vi "MultiPAS-UV.vi"() -> ()   [LabVIEW 2011]
uses:
  sub/crd/fit/Analysis/analys_meth.ctl
  <vilib>/Analysis/4window.llb/windowTd.ctl
  sub/saveBuildHeader_III.vi
  <vilib>/Utility/file.llb/Write To Spreadsheet File (string).vi
  sub/laserDiagnose_UV.vi
  <vilib>/Instr/_visa.llb/VISA Configure Serial Port (Instr).vi
  sub/QMH/QMH Add Message to Queue (Single Element).vi
  sub/absCalcPlot_UV.vi
  <vilib>/measure/maspectr.llb/FFT Spectrum (Mag-Phase) for 1 Chan.vi
  sub/fftGetMags.vi
  sub/rollingAverage_III.vi
  sub/micUnbundle_III.vi
  sub/pdNormalize_III.vi
  sub/QMH/QMH Add Message to Queue (Array).vi
  <vilib>/measure/NI_MAPro.lvlib
  <vilib>/Analysis/NI_AALPro.lvlib
panel:
  out "working directory":path
  in  "No. Averages":i32=16
  out "saveString":string
  in  "Save Average":bool
  out "Chopper On":bool=TRUE caption="Overtemp"
  in  "Chopper":bool=TRUE
  out "PAS Save":bool caption="Overtemp"
  in  "Data 2":i32[][](array[numeric])=[[-16374, -7248, 2543, 12030, 20279, 26487, 30037, 30583, 28073, 22744, 15131, 5976, -3818, -13288, -21504, -27663, -31155, -31636, -29064, -23686, -16036, -6862, 2936, 12388, 20571, 26684, 30122, 30546, 27911, 22483, 14793, 5595, -4207, -13644, -21795, -27855, -31232, -31591, -28898, -23423, -15695, -6476, 3323, 12743, 20858, 26873, 30194, 30492, 27744, 22213, 14447, 5207, -4597, -14002, -22082, -28044, -31304, -31540, -28731, -23149, -15348, -6093, 3713, 13101, 21145, 27063, 30265, 30442, 27576, 21943, 14103, 4822, -4984, -14354, -22365, -28230, -31373, -31485, -28556, -22876, -14998, -5702, 4104, 13452, 21428, 27245, 30335, 30388, 27400, 21669, 13754, 4435, -5375, -14705, -22643, -28407, -31436, -31426, -28378, -22598, -14648, -5314, 4497, 13803, 21706, 27423, 30394, 30325, 27221, 21390, 13402, 4045, -5763, -15056, -22921, -28586, -31496, -31361, -28198, -22319, -14297, -4924, 4879, 14151, 21982, 27597, 30451, 30257, 27038, 21107, 13050, 3658, -6149, -15402, -23193, -28754, -31546, -31290, -28010, -22033, -13944, -4536, 5266, 14498, 22252, 27767, 30500, 30184, 26849, 20821, 12696, 3267, -6535, -15748, -23462, -28924, -31596, -31216, -27821, -21748, -13587, -4147, 5653, 14838, 22519, 27930, 30549, 30110, 26658, 20535, 12337, 2878, -6919, -16089, -23727, -29087, -31641, -31137, -27627, -21457, -13229, -3753, 6038, 15181, 22786, 28093, 30591, 30031, 26461, 20243, 11979, 2485, -7303, -16428, -23991, -29244, -31678, -31053, -27426, -21159, -12867, -3360, 6424, 15524, 23043, 28252, 30633, 29946, 26262, 19946, 11617, 2096, -7686, -16764, -24246, -29398, -31712, -30964, -27224, -20862, -12503, -2971, 6803, 15859, 23301, 28401, 30661, 29852, 26058, 19648, 11254, 1703, -8069, -17099, -24500, -29547, -31741, -30870, -27018, -20562, -12138, -2575, 7188, 16192, 23556, 28549, 30689, 29756, 25848, 19348, 10891, 1312, -8448, -17430, -24753, -29691, -31765, -30773, -26806, -20259, -11775, -2186, 7566, 16521, 23801, 28690, 30709, 29656, 25634, 19038, 10523, 919, -8831, -17762, -24997, -29833, -31788, -30672, -26593, -19955, -11409, -1792, 7944, 16850, 24047, 28830, 30724, 29548, 25416, 18729, 10152, 523, -9212, -18092, -25245, -29969, -31805, -30566, -26375, -19647, -11041, -1403, 8319, 17173, 24287, 28963, 30734, 29436, 25192, 18418, 9781, 130, -9587, -18413, -25481, -30101, -31814, -30449, -26150, -19332, -10666, -1007, 8697, 17497, 24524, 29090, 30745, 29325, 24968, 18105, 9408, -263, -9962, -18735, -25718, -30228, -31820, -30334, -25921, -19016, -10296, -618, 9072, 17814, 24756, 29213, 30746, 29202, 24738, 17787, 9036, -657, -10338, -19058, -25951, -30350, -31818, -30214, -25690, -18699, -9922, -224, 9442, 18128, 24984, 29330, 30738, 29078, 24502, 17466, 8658, -1050, -10710, -19371, -26178, -30467, -31814, -30088, -25458, -18382, -9550, 167, 9812, 18440, 25206, 29443, 30732, 28947, 24264, 17143, 8281, -1445, -11083, -19685, -26404, -30581, -31807, -29959, -25221, -18059, -9175, 556, 10178, 18750, 25426, 29548, 30718, 28809, 24018, 16812, 7901, -1842, -11457, -19996, -26624, -30690, -31795, -29824, -24980, -17733, -8799, 950, 10549, 19058, 25643, 29655, 30700, 28673, 23773, 16484, 7523, -2235, -11824, -20304, -26840, -30793, -31772, -29682, -24731, -17402, -8415, 1341, 10916, 19363, 25856, 29755, 30677, 28528, 23522, 16151, 7141, -2626, -12191, -20607, -27051, -30891, -31746, -29536, -24481, -17070, -8035, 1733, 11280, 19664, 26064, 29851, 30648, 28381, 23272, 15818, 6762, -3019, -12555, -20906, -27258, -30984, -31717, -29391, -24226, -16736, -7655, 2128, 11641, 19962, 26270, 29940, 30615, 28229, 23013, 15483, 6376, -3409, -12914, -21204, -27459, -31071, -31684, -29236, -23967, -16398, -7271, 2515, 12005, 20258, 26468, 30024, 30577, 28072, 22753, 15143, 5990, -3802, -13276, -21497, -27660, -31157, -31643, -29076, -23707, -16058, -6886, 2908, 12363, 20550, 26666, 30107, 30536, 27914, 22489, 14805, 5607, -4192, -13633, -21787, -27849, -31230, -31597, -28911, -23438, -15716, -6501, 3298, 12719, 20839, 26858, 30182, 30488, 27744, 22223, 14459, 5225, -4579, -13988, -22071, -28040, -31304, -31549, -28743, -23167, -15368, -6113, 3693, 13076, 21126, 27047, 30255, 30438, 27576, 21950, 14113, 4837, -4971, -14340, -22354, -28224, -31375, -31494, -28570, -22895, -15022, -5725, 4080, 13430, 21408, 27230, 30324, 30384, 27402, 21676, 13766, 4449, -5360, -14694, -22636, -28409, -31440, -31436, -28397, -22617, -14674, -5338, 4467, 13781, 21686, 27408, 30385, 30320, 27224, 21398, 13418, 4062, -5748, -15044, -22913, -28584, -31498, -31368, -28212, -22339, -14321, -4948, 4856, 14131, 21963, 27583, 30440, 30254, 27042, 21118, 13062, 3669, -6137, -15390, -23183, -28751, -31551, -31297, -28024, -22049, -13962, -4556, 5245, 14476, 22235, 27754, 30497, 30186, 26857, 20834, 12710, 3283, -6519, -15733, -23453, -28921, -31600, -31226, -27837, -21765, -13610, -4168, 5628, 14820, 22502, 27918, 30540, 30109, 26664, 20544, 12354, 2891, -6906, -16074, -23719, -29085, -31646, -31148, -27642, -21475, -13251, -3777, 6014, 15160, 22765, 28078, 30583, 30027, 26468, 20251, 11994, 2501, -7292, -16415, -23980, -29242, -31682, -31064, -27443, -21181, -12892, -3386, 6397, 15501, 23026, 28238, 30624, 29944, 26269, 19959, 11633, 2110, -7673, -16753, -24239, -29395, -31719, -30974, -27239, -20882, -12528, -2993, 6782, 15835, 23285, 28390, 30651, 29852, 26063, 19660, 11271, 1720, -8053, -17087, -24493, -29546, -31746, -30880, -27031, -20583, -12163, -2599, 7166, 16173, 23538, 28538, 30684, 29758, 25853, 19356, 10906, 1327, -8433, -17416, -24743, -29688, -31769, -30782, -26821, -20280, -11797, -2208, 7543, 16501, 23786, 28680, 30704, 29656, 25642, 19053, 10540, 936, -8814, -17747, -24989, -29827, -31787, -30678, -26606, -19973, -11430, -1817, 7923, 16829, 24031, 28819, 30721, 29552, 25424, 18746, 10174, 543, -9191, -18072, -25231, -29962, -31802, -30567, -26384, -19660, -11057, -1422, 8302, 17159, 24274, 28952, 30738, 29443, 25205, 18435, 9801, 150, -9568, -18401, -25472, -30095, -31811, -30457, -26163, -19349, -10687, -1031, 8679, 17481, 24511, 29082, 30742, 29327, 24979, 18121, 9431, -241, -9943, -18717, -25707, -30221, -31815, -30337, -25930, -19029, -10312, -631, 9058, 17802, 24745, 29207, 30746, 29209, 24750, 17805, 9057, -634, -10316, -19037, -25937, -30340, -31814, -30217, -25700, -18713, -9939, -240, 9429, 18117, 24976, 29328, 30740, 29088, 24519, 17486, 8682, -1027, -10688, -19352, -26164, -30458, -31810, -30091, -25465, -18390, -9561, 154, 9800, 18433, 25201, 29442, 30735, 28959, 24282, 17165, 8308, -1420, -11063, -19665, -26386, -30570, -31801, -29961, -25227, -18068, -9185, 547, 10171, 18745, 25424, 29552, 30726, 28825, 24038, 16835, 7925, -1815, -11429, -19974, -26608, -30681, -31789, -29826, -24984, -17741, -8807, 938, 10536, 19047, 25636, 29657, 30708, 28685, 23794, 16510, 7550, -2205, -11798, -20280, -26821, -30782, -31766, -29684, -24737, -17411, -8429, 1331, 10906, 19356, 25851, 29758, 30684, 28544, 23546, 16178, 7169, -2598, -12162, -20582, -27035, -30879, -31744, -29540, -24485, -17080, -8048, 1721, 11267, 19655, 26061, 29852, 30654, 28395, 23291, 15843, 6786, -2993, -12527, -20884, -27240, -30974, -31713, -29390, -24230, -16744, -7662, 2115, 11635, 19957, 26268, 29945, 30624, 28246, 23035, 15509, 6406, -3382, -12889, -21180, -27444, -31061, -31677, -29236, -23975, -16408, -7284], [-19329, -1252, 17344, 29341, 30145, 19451, 1353, -17227, -29174, -29920, -19175, -1056, 17506, 29408, 30095, 19300, 1159, -17387, -29238, -29860, -19019, -860, 17671, 29475, 30037, 19143, 960, -17553, -29307, -29809, -18866, -664, 17832, 29545, 29987, 18991, 771, -17707, -29365, -29749, -18707, -466, 17992, 29605, 29926, 18832, 570, -17873, -29434, -29694, -18556, -272, 18151, 29670, 29869, 18676, 375, -18031, -29495, -29633, -18395, -75, 18310, 29729, 29809, 18516, 175, -18194, -29561, -29579, -18238, 120, 18469, 29792, 29750, 18362, -17, -18347, -29617, -29515, -18076, 316, 18629, 29848, 29682, 18197, -218, -18510, -29679, -29456, -17921, 513, 18787, 29910, 29626, 18042, -408, -18664, -29734, -29388, -17757, 709, 18941, 29965, 29560, 17875, -609, -18823, -29791, -29326, -17600, 904, 19095, 30023, 29495, 17717, -802, -18975, -29845, -29260, -17434, 1099, 19251, 30075, 29425, 17551, -1001, -19131, -29901, -29194, -17277, 1296, 19408, 30130, 29359, 17393, -1193, -19284, -29953, -29124, -17112, 1491, 19560, 30184, 29290, 17225, -1392, -19440, -30008, -29056, -16949, 1686, 19713, 30237, 29226, 17069, -1581, -19587, -30054, -28982, -16781, 1883, 19866, 30287, 29151, 16898, -1781, -19742, -30107, -28913, -16616, 2079, 20018, 30337, 29082, 16737, -1973, -19888, -30152, -28838, -16449, 2275, 20167, 30383, 29006, 16564, -2174, -20041, -30200, -28765, -16282, 2471, 20321, 30430, 28934, 16403, -2364, -20187, -30243, -28688, -16113, 2669, 20465, 30470, 28853, 16230, -2568, -20341, -30294, -28618, -15953, 2860, 20615, 30519, 28783, 16070, -2755, -20486, -30335, -28537, -15779, 3057, 20760, 30560, 28700, 15892, -2956, -20637, -30378, -28461, -15613, 3252, 20909, 30605, 28628, 15730, -3145, -20777, -30418, -28377, -15440, 3446, 21054, 30645, 28543, 15557, -3345, -20927, -30460, -28299, -15271, 3643, 21199, 30686, 28465, 15391, -3534, -21066, -30495, -28215, -15100, 3839, 21345, 30722, 28380, 15214, -3734, -21213, -30534, -28134, -14928, 4032, 21487, 30760, 28300, 15044, -3926, -21355, -30570, -28052, -14757, 4225, 21627, 30792, 28209, 14870, -4123, -21501, -30607, -27968, -14586, 4419, 21768, 30832, 28129, 14702, -4314, -21637, -30639, -27880, -14413, 4612, 21907, 30859, 28040, 14521, -4515, -21780, -30675, -27796, -14241, 4804, 22048, 30895, 27953, 14352, -4702, -21919, -30705, -27707, -14064, 4999, 22187, 30922, 27859, 14172, -4900, -22060, -30739, -27620, -13892, 5193, 22326, 30954, 27773, 14003, -5090, -22194, -30765, -27524, -13712, 5386, 22462, 30981, 27679, 13823, -5285, -22333, -30794, -27436, -13538, 5580, 22600, 31013, 27591, 13650, -5476, -22466, -30820, -27343, -13363, 5770, 22732, 31033, 27491, 13468, -5673, -22605, -30848, -27251, -13187, 5964, 22870, 31060, 27401, 13292, -5863, -22736, -30870, -27155, -13010, 6156, 23000, 31079, 27299, 13111, -6058, -22873, -30895, -27060, -12833, 6347, 23134, 31104, 27208, 12936, -6248, -23004, -30918, -26965, -12652, 6536, 23260, 31120, 27106, 12753, -6444, -23136, -30939, -26865, -12472, 6729, 23395, 31148, 27011, 12578, -6634, -23266, -30959, -26766, -12296, 6919, 23523, 31161, 26907, 12392, -6830, -23402, -30982, -26665, -12115, 7109, 23652, 31180, 26809, 12213, -7016, -23524, -30992, -26564, -11932, 7301, 23777, 31195, 26704, 12032, -7210, -23655, -31011, -26464, -11755, 7492, 23907, 31211, 26605, 11855, -7395, -23778, -31024, -26358, -11573, 7680, 24031, 31218, 26494, 11665, -7592, -23908, -31039, -26258, -11392, 7871, 24158, 31237, 26394, 11491, -7775, -24031, -31050, -26153, -11210, 8063, 24281, 31247, 26285, 11302, -7972, -24159, -31062, -26046, -11027, 8250, 24407, 31258, 26180, 11124, -8157, -24276, -31067, -25937, -10841, 8438, 24526, 31265, 26071, 10936, -8347, -24401, -31078, -25829, -10659, 8630, 24649, 31275, 25965, 10755, -8533, -24522, -31087, -25721, -10474, 8816, 24770, 31280, 25853, 10566, -8726, -24641, -31091, -25608, -10290, 9003, 24891, 31287, 25746, 10386, -8910, -24756, -31095, -25498, -10105, 9192, 25008, 31287, 25627, 10196, -9102, -24881, -31101, -25386, -9919, 9381, 25127, 31296, 25521, 10019, -9284, -24994, -31099, -25268, -9732, 9570, 25243, 31293, 25403, 9826, -9476, -25113, -31105, -25157, -9544, 9756, 25359, 31298, 25291, 9645, -9655, -25225, -31099, -25040, -9359, 9942, 25473, 31291, 25167, 9453, -9847, -25341, -31102, -24926, -9173, 10124, 25586, 31294, 25057, 9269, -10029, -25450, -31095, -24809, -8986, 10310, 25696, 31284, 24931, 9078, -10218, -25564, -31094, -24688, -8798, 10497, 25812, 31287, 24819, 8896, -10399, -25673, -31085, -24567, -8608, 10682, 25922, 31278, 24698, 8703, -10587, -25785, -31080, -24448, -8422, 10866, 26033, 31274, 24582, 8522, -10765, -25890, -31067, -24321, -8230, 11050, 26140, 31263, 24455, 8325, -10952, -26001, -31064, -24201, -8040, 11234, 26248, 31255, 24338, 8142, -11132, -26106, -31054, -24079, -7852, 11417, 26353, 31243, 24207, 7948, -11316, -26217, -31041, -23952, -7662, 11601, 26464, 31236, 24089, 7763, -11494, -26315, -31025, -23829, -7471, 11782, 26562, 31217, 23957, 7567, -11682, -26422, -31014, -23702, -7282, 11962, 26667, 31205, 23834, 7383, -11859, -26521, -30998, -23575, -7092, 12144, 26770, 31187, 23704, 7186, -12043, -26626, -30981, -23444, -6900, 12328, 26875, 31176, 23582, 7003, -12218, -26724, -30962, -23316, -6709, 12505, 26971, 31154, 23446, 6805, -12401, -26825, -30946, -23189, -6517, 12687, 27073, 31139, 23322, 6620, -12576, -26919, -30922, -23054, -6323, 12867, 27170, 31114, 23185, 6422, -12760, -27022, -30904, -22923, -6132, 13047, 27272, 31096, 23060, 6237, -12934, -27114, -30879, -22790, -5940, 13222, 27362, 31068, 22921, 6041, -13116, -27212, -30855, -22657, -5748, 13401, 27461, 31048, 22790, 5853, -13289, -27302, -30828, -22522, -5555, 13577, 27549, 31019, 22652, 5652, -13472, -27398, -30806, -22388, -5362, 13753, 27645, 30995, 22521, 5463, -13642, -27487, -30776, -22248, -5169, 13928, 27733, 30963, 22376, 5266, -13823, -27584, -30750, -22113, -4975, 14106, 27828, 30937, 22246, 5082, -13992, -27669, -30717, -21974, -4782, 14280, 27914, 30902, 22101, 4880, -14174, -27760, -30689, -21837, -4588, 14454, 28006, 30875, 21965, 4692, -14340, -27843, -30653, -21693, -4391, 14631, 28092, 30840, 21822, 4494, -14519, -27934, -30620, -21552, -4198, 14805, 28179, 30808, 21688, 4308, -14687, -28015, -30582, -21410, -4004, 14975, 28262, 30770, 21540, 4106, -14861, -28103, -30548, -21268, -3808, 15149, 28349, 30739, 21402, 3916, -15032, -28183, -30512, -21124, -3614, 15319, 28430, 30697, 21255, 3715, -15205, -28267, -30475, -20982, -3421, 15490, 28513, 30664, 21116, 3524, -15376, -28348, -30435, -20837, -3225, 15660, 28592, 30617, 20962, 3327, -15550, -28432, -30397, -20695, -3032, 15829, 28673, 30581, 20820, 3134, -15711, -28506, -30353, -20546, -2837, 15994, 28746, 30530, 20669, 2933, -15887, -28585, -30311, -20400, -2641, 16167, 28828, 30496, 20528, 2745, -16052, -28660, -30264, -20248, -2445, 16335, 28901, 30445, 20376, 2544, -16221, -28737, -30219, -20102, -2250, 16505, 28983, 30406, 20231, 2357, -16381, -28808, -30171, -19950, -2053, 16670, 29053, 30355, 20075, 2154, -16552, -28883, -30127, -19803, -1859, 16835, 29128, 30308, 19930, 1965, -16714, -28952, -30073, -19650, -1663, 17001, 29192, 30255, 19772, 1764, -16881, -29028, -30026, -19496, -1467, 17165, 29268, 30208, 19626, 1572, -17043, -29095, -29977, -19346]]
  out "Filtering":bool caption="Time has Elapsed"
  in  "Switch Filter":bool
  in  "Auto Filter":bool
  out "Elapsed Time (min)":dbl caption="Elapsed Time (s)" format="%#.1g"
  in  "Filter Length (min)":dbl=6.0 caption="Time Target (s)"
  in  "Sample Length (min)":dbl=24.0 caption="Time Target (s)" format="%#.1f"
  out "Time has Elapsed":bool
  in  "Time Target (s)":dbl=1.0
  in  "All Emit":bool
  in  "Alignment Mode":bool
  in  "445 Emission":bool
  in  "445 Power (mW)":dbl(slide)=75.0 min=0.0 max=75.0 step=1.0 scale=0.0..75.0
  in  "375 Emission":bool
  in  "375 Power (mW)":dbl(slide)=100.0 min=0.0 max=50.0 step=1.0 scale=0.0..50.0
  in  "320 Emission":bool=TRUE
  out "Overtemp":bool
  in  "Tab Control":T1(tab)=enum."Oscilloscope"
  out "Laser Currents":T2(graph)
  in  "Chopper Port":refnum<visa-resource-name>="COM6"
  out "sweeps":path caption="Microphone File Path"
  in  "save interval (ms)":u32=1000
  out "Error Console":T3
  out "pas":path caption="Microphone File Path"
  out "Laser Temperatures":T2(graph)
  in  "pd id":u32=2
  in  "mic id":u32
  in  "mic cal, scu":dbl=5.41531278804282e-05 format="%#_3e"
  in  "mic cal, scu":dbl=5.59307241877627e-05 format="%#_3e"
  in  "320 Port":refnum<visa-resource-name>="COM7"
  in  "375 Port":refnum<visa-resource-name>="COM8"
  in  "445 Port":refnum<visa-resource-name>="COM9"
  in  "Teensy Port":refnum<visa-resource-name>="COM10"
  in  "Save Data":bool
  in  "405 PD Cal 3":dbl=0.0075
  in  "532 PD Cal 3":dbl=0.0861
  in  "660 PD Cal 3":dbl=0.005
  out "Laser Powers":T2(graph)
  in  "tau Rolling Avg":i32=8
  out "error out":errorcluster
  in  "Channel B Settings":T4={"Enabled"=TRUE, "Coupling"=1, "Range"=8, "Analogue Offset"=0.0} {"Range" items=["20 mV"=1, "50 mV"=2, "100 mV"=3, "200 mV"=4, "500 mV"=5, "1 V"=6, "2 V"=7, "5 V"=8, "10 V"=9, "20 V"=10]; "Coupling" items=["AC", "DC"]}
  in  "Rapid Block Acquisition Settings":T5={"preTriggerSamples"=0, "postTriggerSamples"=45000, "timebase"=1, "Down-Sample Mode"=4, "Down Sample Ratio"=10, "Oversample"=1, "Number of Captures"=100} {"Down Sample Ratio" min=1 step=1; "Down-Sample Mode" items=["None"=0, "Aggregate"=1, "Decimate"=2, "Average"=4]}
  in  "crd delay":u32=1000
  in  "Trigger Settings":T6={"Trigger Enabled"=TRUE, "Trigger Source"=enum."Channel B", "Trigger Threshold (Volts)"=1.0, "Trigger Direction"=3, "Trigger Delay (samples)"=0, "Auto Trigger Time (ms)"=1000} {"Trigger Direction" items=["Rising"=2, "Falling"=3]}
  in  "Channel A Settings":T4={"Enabled"=TRUE, "Coupling"=0, "Range"=3, "Analogue Offset"=0.0} {"Range" items=["20 mV"=1, "50 mV"=2, "100 mV"=3, "200 mV"=4, "500 mV"=5, "1 V"=6, "2 V"=7, "5 V"=8, "10 V"=9, "20 V"=10]; "Coupling" items=["AC", "DC"]}
  in  "factor":sgl=10.0
  in  "N":i32=4400
  in  "sweep":bool
  out "freqscan":cluster{i32[], "Best Gaussian Fit":dbl[]}[](graph) caption="Frequency Sweep"
  out "sweep progress":dbl(slide) scale=0.0..1.0
  in  "Autosweep?":bool=TRUE
  in  "set freqs":bool
  out "Calculated Resonance (Hz)":dbl=1370.0
  in  "Data Start Frequency (Hz)":i32=1355
  in  "Data End Frequency (Hz)":i32=1405
  in  "320 F (Hz)":i32=1368
  in  "375 F (Hz)":i32=1372
  in  "445 F (Hz)":i32=1370
  in  "Chart Rolling Average":i32=16
  out "pdwave":waveform(i32)(graph) caption="Photodiode Waveform"
  out "pd ts":cluster{dbl, dbl, dbl}(graph)
  out "pdfft":cluster{"f0":dbl, "df":dbl, "magnitude":dbl[]}(graph) caption="Photodiode FFT"
  in  "rollavg":i32=16 caption="Dispaly Averaging (Transfers to Absorption Data!)"
  out "mic ts":T7(graph)
  out "micfft":cluster{"f0":dbl, "df":dbl, "magnitude":dbl[]}(graph) caption="Photodiode FFT"
  out "micwave":waveform(i32)(graph) caption="Photodiode Waveform"
  in  "tau0":dbl
  in  "getbkg":bool
  out "AAE":dbl(graph)
  in  "Bkg Values (mV)":cluster{dbl, dbl, dbl}
  out "Absorption Spectrum":cluster{dbl[], "Best Power Fit":dbl[]}[](graph)
  in  "cellcal":dbl=95000.0 caption="Cell Calibration Coefficient (mV/mW)"
  out "abs/ext":cluster{dbl, dbl, dbl, "b_ext (1/Mm)":dbl}(graph)
  out "tau":dbl(graph)
  out "decay":cluster{i32, sgl, dbl[]}[](graph)
  out "residual":cluster{i32, sgl, dbl[]}(graph)
  out "Status":string
  in  "Exit":bool
  in  "State Variables":cluster{"CurrentFile":path}
  # "MultiPAS-UV | AeroSmith Labs (2017)"
  # "Laser Control"
  # "Filter Control"
  # "Communications"
  # "Sound Card Parameters"
  # "Data File Options"
  # "File paths are populated automatically at <...\\My Documents\\MultiPAS Data\\>.  To save in another location, turn on \"Save Data\" and follow the prompts to choose an alternate working directory."
  # "Photodiode Calibration"
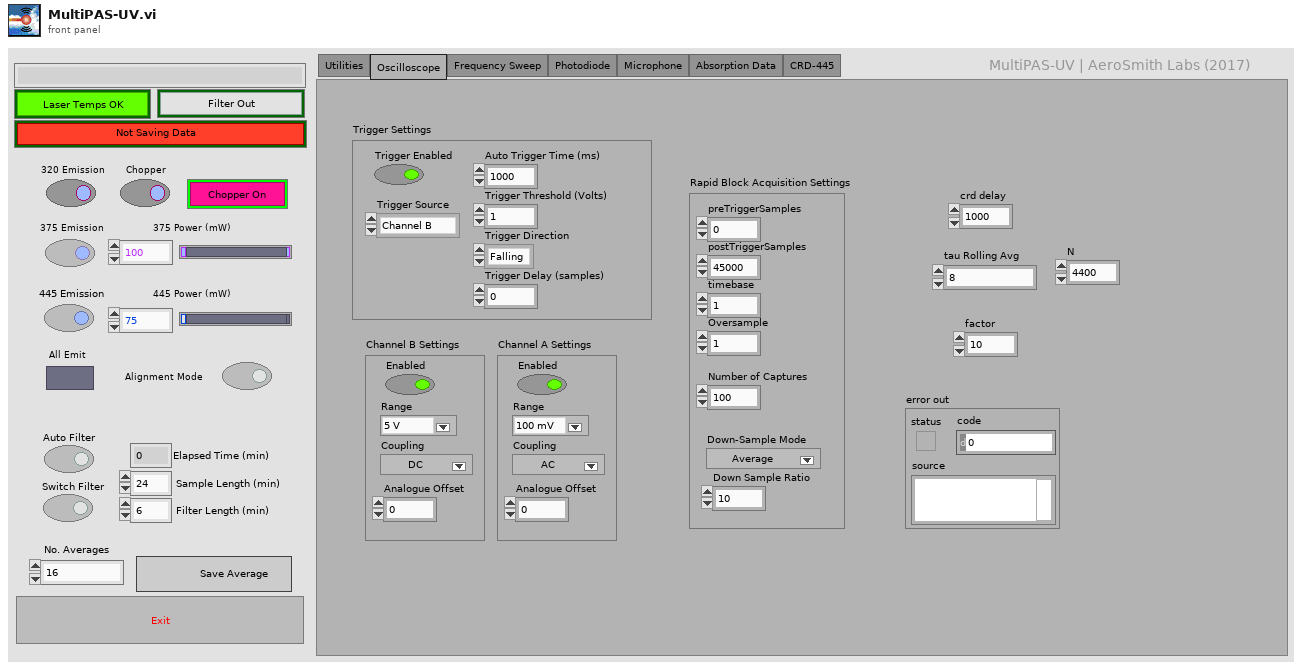
[diagram p1: front panel]
types:
  T1 = enum32{"Utilities", "Oscilloscope", "Frequency Sweep", "Photodiode", "Microphone", "Absorption Data", "CRD-445"}
  T2 = cluster{"Temp (C)":dbl, "Temp (C)":dbl, "Temp (C)":dbl}
  T3 = cluster{"status":bool, "code":i32, "Message":string}
  T4 = cluster{"Enabled":bool, "Coupling":i16, "Range":u16, "Analogue Offset":sgl}
  T5 = cluster{"preTriggerSamples":u32, "postTriggerSamples":u32, "timebase":u32, "Down-Sample Mode":i32, "Down Sample Ratio":u32, "Oversample":i16, "Number of Captures":u32}
  T6 = cluster{"Trigger Enabled":bool, "Trigger Source":enum16{"Channel A", "Channel B", "Channel C", "Channel D", "Ext."}, "Trigger Threshold (Volts)":dbl, "Trigger Direction":u16, "Trigger Delay (samples)":u32, "Auto Trigger Time (ms)":i16}
  T7 = cluster{"422 Mean":dbl, "532 Mean":dbl, "785 Mean":dbl}
  T8 = cluster{"# buffers":i32, "Buffer size":i32, "unit (ms)":enum16{"time (ms)", "Samples"}}
  T9 = typedef "SoundHandle.ctl" = cluster{"DeviceID":u16, "Samples/buf":u32, "Sampl rate":u32, "Bits/sample":u16, "Channels":u8, "Opened":bool}
  T10 = cluster{"Output Power at Laser Head":dbl, "Output Power at Laser Head":dbl, "Output Power at Laser Head":dbl}
  T11 = cluster{"Current (mA)":dbl, "Current (mA)":dbl, "Current (mA)":dbl}
  T12 = cluster{"405 Mean":dbl, "532 Mean":dbl, "660 Mean":dbl}
  T13 = typedef "NI_AALPro.lvlib/windowTd.ctl" = u32
  T14 = cluster{"785 New Array":dbl[], "785 Mean":dbl, "785 SD":dbl}
  T15 = cluster{"532 New Array":dbl[], "532 Mean":dbl, "532 SD":dbl}
  T16 = cluster{"422 New Array":dbl[], "422 Mean":dbl, "422 SD":dbl}
  T17 = typedef "analys_meth.ctl" = enum16{"DFT-1", "DFT-5", "LRS"}
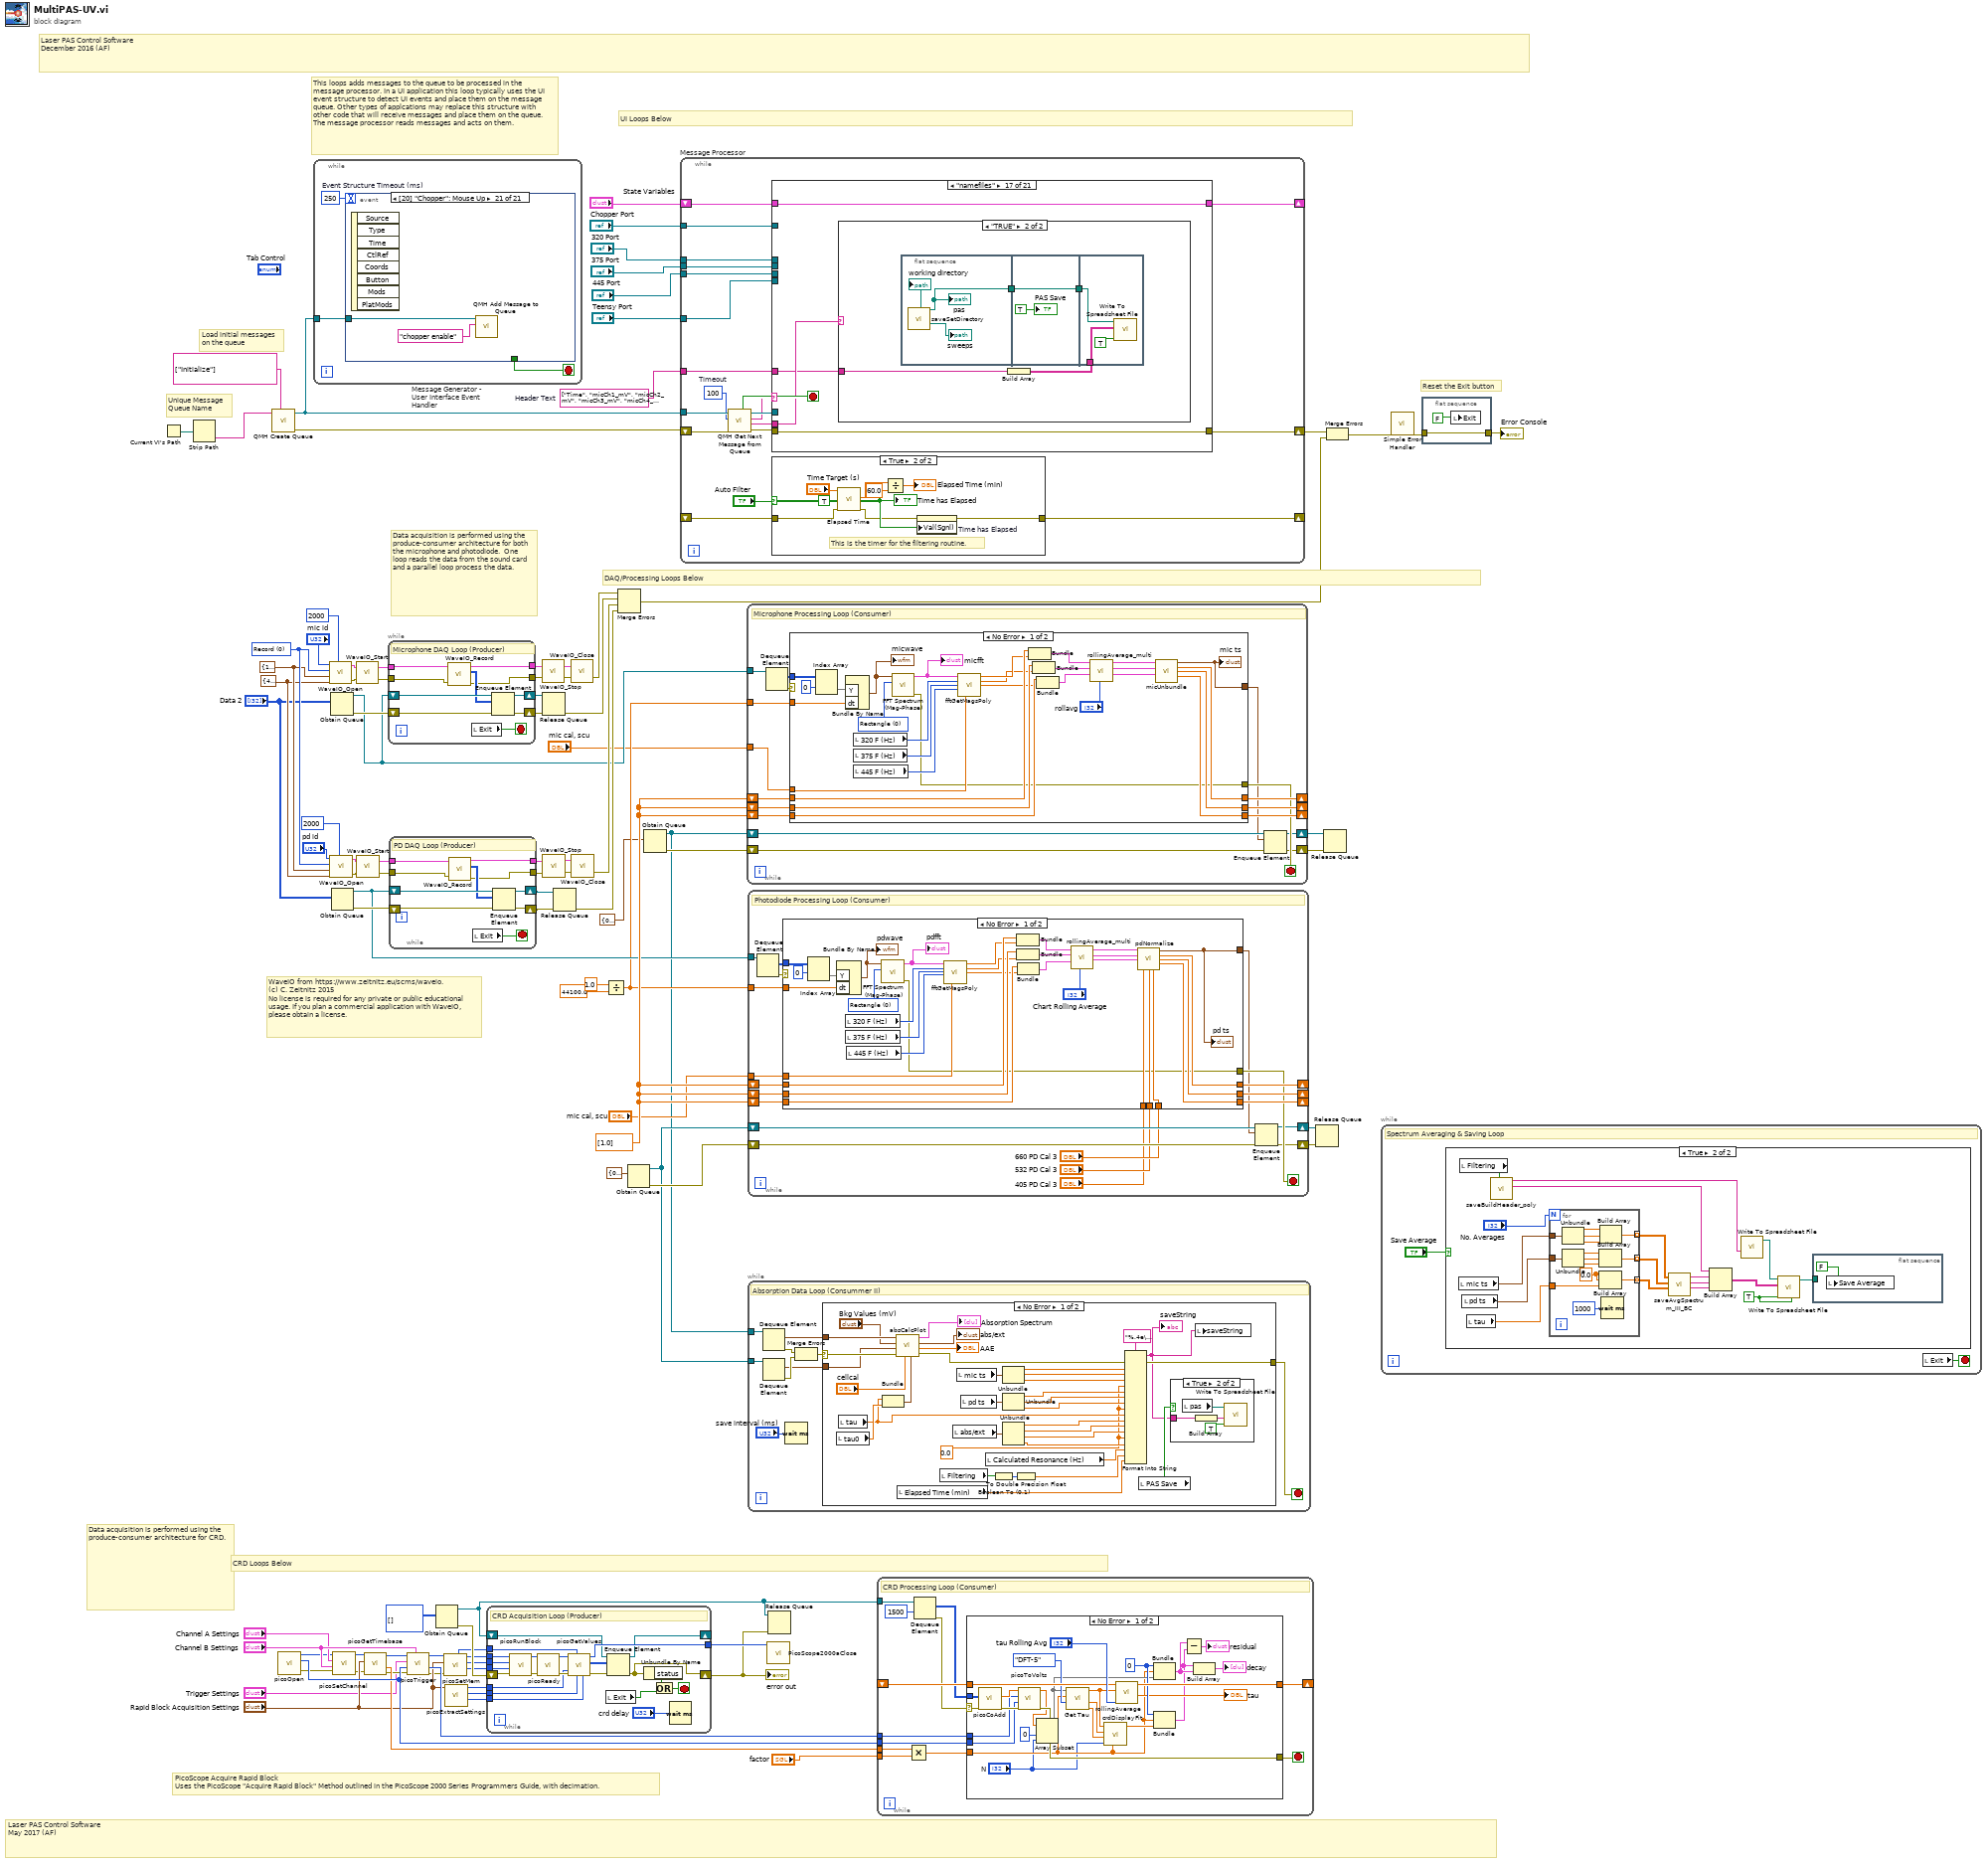
[diagram p0: block diagram]
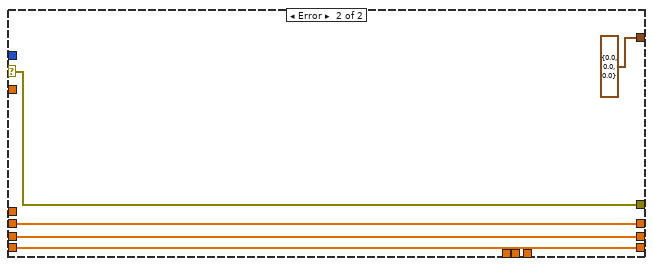
[diagram p6: hidden frame]
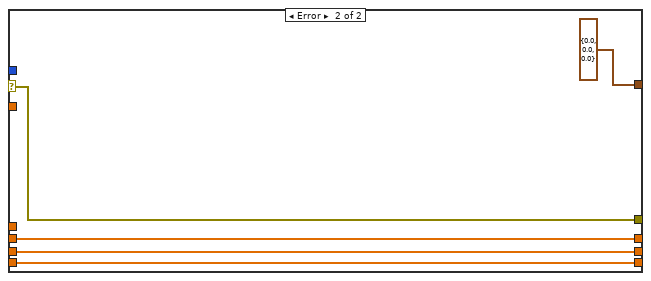
[diagram p7: hidden frame]
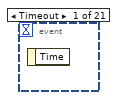
[diagram p8: hidden frame]
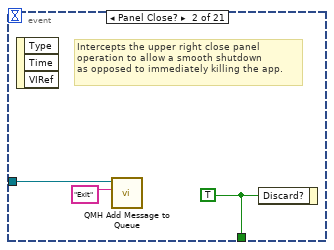
[diagram p9: hidden frame]
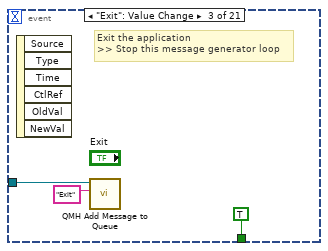
[diagram p10: hidden frame]
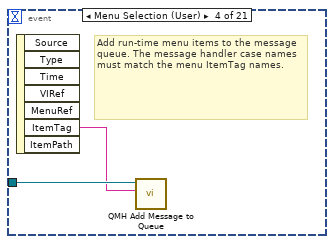
[diagram p11: hidden frame]
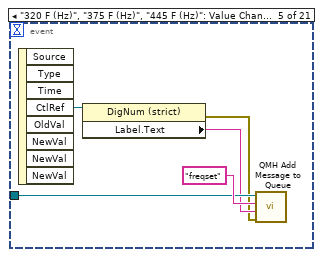
[diagram p12: hidden frame]
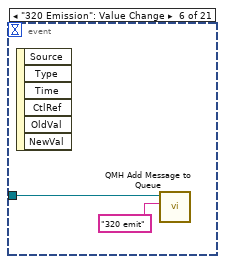
[diagram p13: hidden frame]
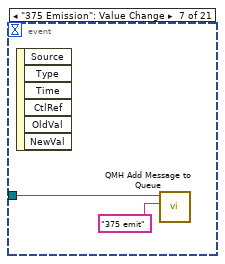
[diagram p14: hidden frame]
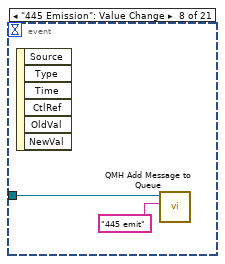
[diagram p15: hidden frame]
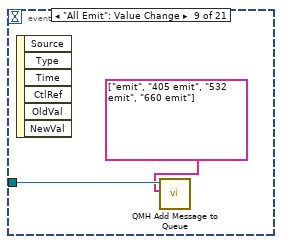
[diagram p16: hidden frame]
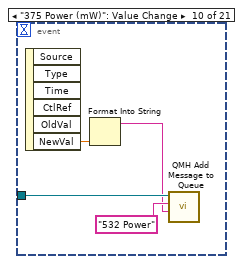
[diagram p17: hidden frame]
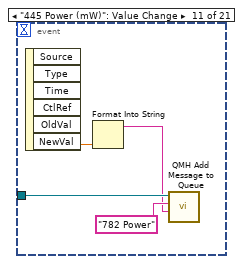
[diagram p18: hidden frame]
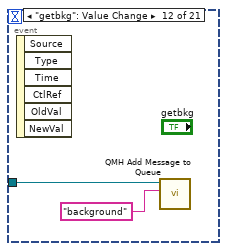
[diagram p19: hidden frame]
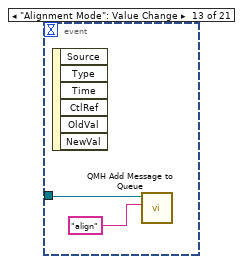
[diagram p20: hidden frame]
diagram:
  w30 = string[] ["Time", "micCh1_mV", "micCh2_mV", "micCh3_mV", "micCh4_mV", "pdCh1_mV", "pdCh2_mV", "pdCh3_mV", "pdCh4_mV", "tau_sec", "babsCh1_Mm", "babsCh2_Mm", "babsCh3_Mm", "babsCh4_Mm", "bext_Mm", "fres_Hz", "filter_state", "elapsedTime_min"]  # Header Text
  w50 = T8 {"# buffers"=10, "Buffer size"=44100, "unit (ms)"=enum."Samples"} ("Buffer")
  w49 = cluster{"Rate":i32, "Bits":i32, "Channels":i32} {"Rate"=44100, "Bits"=24, "Channels"=2} ("Format")
  w51 = u16 0 items=["Record", "Play", "Loopback", "ASIO input", "ASIO output"] ("Direction (Record)")
  w81 = dbl[] [1.0] ("X")
  # "PicoScope Acquire Rapid Block\nUses the PicoScope \"Acquire Rapid Block\" Method outlined in the PicoScope 2000 Series Programmers Guide, with decimation."
  # "Data acquisition is performed using the produce-consumer architecture for CRD."
  # "CRD Loops Below"
  # "Laser PAS Control Software\nMay 2017 (AF)"
  # "Laser PAS Control Software\nDecember 2016 (AF)"
  # "Data acquisition is performed using the produce-consumer architecture for both the microphone and photodiode.  One loop reads the data from the sound card and a parallel loop process the data."
  # "WaveIO from https://www.zeitnitz.eu/scms/waveio.\n(c) C. Zeitnitz 2015\nNo license is required for any private or public educational usage. If you plan a commercial application with WaveIO, please obtain a license."
  # "This loops adds messages to the queue to be processed in the message processor. In a UI application this loop typically uses the UI event structure to detect UI events and place them on the message queue. Other types of applcations may replace this structure with other code that will receive messages and place them on the queue.  The message processor reads messages and acts on them."
  # "Reset the Exit button"
  # "Unique Message\nQueue Name"
  # "Load initial messages\non the queue"
  # "DAQ/Processing Loops Below"
  # "UI Loops Below"
  n1 = Current VI's Path() -> (path=w96:path)
  n2 = Strip Path(path=w96) -> (name=w97:string)  [unwired: 1 out]
  n3 = call "QMH Create Queue.vi"("Initial Messages"=string[] ["Initialize"], "Message queue name (unnamed)"=w97) -> ("error out"=w93:errorcluster, "queue out"=w78:refnum<queue>)  [unwired: 8 in]
  n4 = call "picoOpen.vi"() -> ("error out"=w5:errorcluster, "maxADC"=w24:i16, "Handle Out"=w4:i16)  [unwired: 8 in, 1 out]
  n5 = while "Message Generator - User Interface Event Handler" {
    tunnel: w78 -> [w98]
    stop <- w99 stop-if-true
    w100 = 250  # Event Structure Timeout (ms)
    n6 = event shown="[20] \"Chopper\": Mouse Up" {
      selector: _ -> [_ _ _ _ _ _ _ _ _ _ _ _ _ _ _ _ _ _ _ _ _]
      dyn-events: _ -> [_ _ _ _ _ _ _ _ _ _ _ _ _ _ _ _ _ _ _ _ _]
      timeout: w100 -> [_ _ _ _ _ _ _ _ _ _ _ _ _ _ _ _ _ _ _ _ _]
      tunnel: [_ w103 TRUE ("Discard?") _ _ _ _ _ _ _ _ _ _ _ _ _ _ _ _ _ _] -> w99
      tunnel: w98 -> [_ w102 w105 w108 w112 w114 w116 w118 w121 w124 w128 w130 w132 w135 w139 w144 w149 w153 w158 w160 w162]
      event Timeout {
        n7 = event-data() -> ()  [unwired: 1 in, 1 out]
      }
      event Panel Close? {
        w103 = TRUE ("Discard?")
        # "Intercepts the upper right close panel\noperation to allow a smooth shutdown\nas opposed to immediately killing the app."
        n8 = event-data() -> ()  [unwired: 1 in, 3 out]
        n9 = call-poly "QMH Add Message to Queue.vi"("Message"="Exit", "queue in"=w102) -> ()  [unwired: 8 in, 2 out]
        n10 = event-data("Discard?"=w103) -> ()  [unwired: 1 in, 1 out]
      }
      event "Exit": Value Change {
        # "Exit the application\n>> Stop this message generator loop"
        n11 = event-data() -> ()  [unwired: 1 in, 6 out]
        n12 = call-poly "QMH Add Message to Queue.vi"("Message"="Exit", "queue in"=w105) -> ()  [unwired: 8 in, 2 out]
      }
      event Menu Selection (User) {
        # "Add run-time menu items to the message\nqueue. The message handler case names must match the menu ItemTag names."
        n13 = event-data() -> ("ItemTag"=w107:string)  [unwired: 1 in, 6 out]
        n14 = call-poly "QMH Add Message to Queue.vi"("Message"=w107, "queue in"=w108) -> ()  [unwired: 8 in, 2 out]
      }
      event "320 F (Hz)", "375 F (Hz)", "445 F (Hz)": Value Change {
        n15 = event-data() -> ("CtlRef"=w111:refnum<vi>)  [unwired: 1 in, 7 out]
        n16 = property class="DigNum (strict)"(reference=w111) -> (error out=w109:errorcluster, "Label.Text"=w110:string)  [unwired: 1 in, 1 out]
        n17 = call-poly "QMH Add Message to Queue.vi"("error in (no error)"=w109, "Parameter"=w110, "Message"="freqset", "queue in"=w112) -> ()  [unwired: 6 in, 2 out]
      }
      event "320 Emission": Value Change {
        n18 = event-data() -> ()  [unwired: 1 in, 6 out]
        n19 = call-poly "QMH Add Message to Queue.vi"("Message"="320 emit", "queue in"=w114) -> ()  [unwired: 8 in, 2 out]
      }
      event "375 Emission": Value Change {
        n20 = event-data() -> ()  [unwired: 1 in, 6 out]
        n21 = call-poly "QMH Add Message to Queue.vi"("Message"="375 emit", "queue in"=w116) -> ()  [unwired: 8 in, 2 out]
      }
      event "445 Emission": Value Change {
        n22 = event-data() -> ()  [unwired: 1 in, 6 out]
        n23 = call-poly "QMH Add Message to Queue.vi"("Message"="445 emit", "queue in"=w118) -> ()  [unwired: 8 in, 2 out]
      }
      event "All Emit": Value Change {
        n24 = event-data() -> ()  [unwired: 1 in, 6 out]
        n25 = call-poly "QMH Add Message to Queue.vi"("Messages"=string[] ["emit", "405 emit", "532 emit", "660 emit"], "queue in"=w121) -> ()  [unwired: 8 in, 2 out]
      }
      event "375 Power (mW)": Value Change {
        n26 = event-data() -> ("NewVal"=w123:dbl)  [unwired: 1 in, 5 out]
        n27 = Format Into String(w123) -> (resulting string=w122:string)  [unwired: 3 in, 1 out]
        n28 = call-poly "QMH Add Message to Queue.vi"("Parameter"=w122, "Message"="532 Power", "queue in"=w124) -> ()  [unwired: 7 in, 2 out]
      }
      event "445 Power (mW)": Value Change {
        n29 = event-data() -> ("NewVal"=w127:dbl)  [unwired: 1 in, 5 out]
        n30 = Format Into String(w127) -> (resulting string=w126:string)  [unwired: 3 in, 1 out]
        n31 = call-poly "QMH Add Message to Queue.vi"("Parameter"=w126, "Message"="782 Power", "queue in"=w128) -> ()  [unwired: 7 in, 2 out]
      }
      event "getbkg": Value Change {
        n32 = event-data() -> ()  [unwired: 1 in, 6 out]
        n33 = call-poly "QMH Add Message to Queue.vi"("Message"="background", "queue in"=w130) -> ()  [unwired: 8 in, 2 out]
      }
      event "Alignment Mode": Value Change {
        n34 = event-data() -> ()  [unwired: 1 in, 6 out]
        n35 = call-poly "QMH Add Message to Queue.vi"("Message"="align", "queue in"=w132) -> ()  [unwired: 8 in, 2 out]
      }
      event "sweep": Value Change {
        n36 = event-data() -> ()  [unwired: 1 in, 6 out]
        n37 = call-poly "QMH Add Message to Queue.vi"("Message"="sweep", "queue in"=w135) -> ()  [unwired: 8 in, 2 out]
      }
      event "set freqs": Value Change {
        n38 = event-data() -> ()  [unwired: 1 in, 6 out]
        n39 = local read "Calculated Resonance (Hz)"() -> (w138:dbl)
        n40 = Format Into String(w138) -> (resulting string=w137:string, error out=w136:errorcluster)  [unwired: 3 in]
        n41 = call-poly "QMH Add Message to Queue.vi"("error in (no error)"=w136, "Parameter"=w137, "Message"="setfreqs", "queue in"=w139) -> ()  [unwired: 6 in, 2 out]
      }
      event "Save Data": Value Change {
        n42 = event-data() -> ("NewVal"=w143:bool)  [unwired: 1 in, 5 out]
        n43 = Format Into String(w143) -> (resulting string=w142:string, error out=w141:errorcluster)  [unwired: 3 in]
        n44 = call-poly "QMH Add Message to Queue.vi"("error in (no error)"=w141, "Parameter"=w142, "Message"="namefiles", "queue in"=w144) -> ()  [unwired: 6 in, 2 out]
      }
      event "Switch Filter": Value Change {
        n45 = event-data() -> ("NewVal"=w148:bool)  [unwired: 1 in, 5 out]
        n46 = local write "Filtering"(w148) -> ()
        n47 = Format Into String(w148) -> (resulting string=w146:string)  [unwired: 3 in, 1 out]
        n48 = call-poly "QMH Add Message to Queue.vi"("Parameter"=w146, "Message"="filterswitch", "queue in"=w149) -> ()  [unwired: 7 in, 2 out]
      }
      event "Time has Elapsed": Value Change {
        n49 = event-data() -> ("NewVal"=w152:bool)  [unwired: 1 in, 5 out]
        n50 = local read "Filtering"() -> (w151:bool)
        n51 = call "filterCreateMsg.vi"("time elapsed?"=w152, "auto sweep (true)"="Autosweep?", "filtering (true)"=w151, "queue in"=w153) -> ()  [unwired: 6 in, 2 out]
      }
      event "Calculated Resonance (Hz)": Value Change {
        n52 = event-data() -> ("NewVal"=w156:dbl)  [unwired: 1 in, 5 out]
        n53 = Format Into String(w156) -> (resulting string=w154:string, error out=w155:errorcluster)  [unwired: 3 in]
        n54 = call-poly "QMH Add Message to Queue.vi"("error in (no error)"=w155, "Parameter"=w154, "Message"="setfreqs", "queue in"=w158) -> ()  [unwired: 6 in, 2 out]
      }
      event "PAS Save": Value Change {
        n55 = event-data() -> ()  [unwired: 1 in, 6 out]
        n56 = call-poly "QMH Add Message to Queue.vi"("Message"="setwd", "queue in"=w160) -> ()  [unwired: 8 in, 2 out]
      }
      event "Chopper": Mouse Up {
        n57 = event-data() -> ()  [unwired: 1 in, 8 out]
        n58 = call-poly "QMH Add Message to Queue.vi"("Message"="chopper enable", "queue in"=w162) -> ()  [unwired: 8 in, 2 out]
      }
    }
  }
  n59 = call <userlib>:"WaveIO_Open.vi"("idev"="mic id", "Watchdog timeout (msec) (default=OFF)"=2000, "device type (Record)"=w51, "Buffer Config"=w50, "Format (44kHz, 16Bit, stereo)"=w49) -> ("Sound Handle Out"=w75:T9, "error out"=w74:errorcluster)  [unwired: 2 in]
  n60 = call <userlib>:"WaveIO_Open.vi"("idev"="pd id", "Watchdog timeout (msec) (default=OFF)"=2000, "device type (Record)"=w51, "Buffer Config"=w50, "Format (44kHz, 16Bit, stereo)"=w49) -> ("Sound Handle Out"=w59:T9, "error out"=w60:errorcluster)  [unwired: 2 in]
  n61 = Obtain Queue(element data type="Data 2") -> (queue out=w43:refnum<queue>, error out=w82:errorcluster)  [unwired: 4 in, 1 out]
  n62 = Obtain Queue(element data type="Data 2") -> (queue out=w47:refnum<queue>, error out=w56:errorcluster)  [unwired: 4 in, 1 out]
  n63 = call "picoSetChannel.vi"("error in (no error)"=w5, "Channel B Settings"="Channel B Settings", "Channel A Settings"="Channel A Settings", "Handle Out"=w4) -> ("error out"=w16:errorcluster, "Handle Out"=w19:i16)  [unwired: 6 in]
  n64 = call <userlib>:"WaveIO_Start.vi"("error in (no error)"=w74, "Handle"=w75) -> ("error out"=w72:errorcluster, "Handle Out"=w73:T9)
  n65 = call <userlib>:"WaveIO_Start.vi"("error in (no error)"=w60, "Handle"=w59) -> ("error out"=w62:errorcluster, "Handle Out"=w61:T9)
  n66 = call "picoGetTimebase.vi"("error in (no error)"=w16, "Rapid Block Acquisition Settings"="Rapid Block Acquisition Settings", "handle in"=w19) -> ("error out"=w17:errorcluster, "Sample Interval"=w23:sgl, "handle out"=w18:i16)  [unwired: 6 in]
  n67 = while {
    shift-right: [w171] -> w83
    shift-left: w43 -> [w169]
    shift-right: [w172] -> w84
    shift-left: w82 -> [w170]
    tunnel: w73 -> [w167]
    tunnel: w72 -> [w166]
    tunnel: [w164] -> w69
    tunnel: [w163] -> w68
    stop <- w168 stop-if-true
    # "Microphone DAQ Loop (Producer)"
    n68 = call <userlib>:"WaveIO_Record.vi"("Handle"=w167, "error in (no error)"=w166) -> ("Handle Out"=w164:T9, "Data"=w165:i32[][], "error out"=w163:errorcluster)  [unwired: 1 in, 2 out]
    n69 = local read "Exit"() -> (w168:bool)
    n70 = Enqueue Element(queue=w169, element=w165, error in (no error)=w170) -> (queue out=w171:refnum<queue>, error out=w172:errorcluster)  [unwired: 1 in, 1 out]
  }
  n71 = while {
    shift-right: [w181] -> w55
    shift-left: w47 -> [w179]
    shift-right: [w182] -> w54
    shift-left: w56 -> [w180]
    tunnel: w61 -> [w177]
    tunnel: w62 -> [w176]
    tunnel: [w174] -> w65
    tunnel: [w173] -> w66
    stop <- w178 stop-if-true
    # "PD DAQ Loop (Producer)"
    n72 = call <userlib>:"WaveIO_Record.vi"("Handle"=w177, "error in (no error)"=w176) -> ("Handle Out"=w174:T9, "Data"=w175:i32[][], "error out"=w173:errorcluster)  [unwired: 1 in, 2 out]
    n73 = local read "Exit"() -> (w178:bool)
    n74 = Enqueue Element(queue=w179, element=w175, error in (no error)=w180) -> (queue out=w181:refnum<queue>, error out=w182:errorcluster)  [unwired: 1 in, 1 out]
  }
  n75 = call "picoTrigger.vi"("Trigger Channel Settings"="Channel B Settings", "error in (no error)"=w17, "maxADC"=w24, "Trigger Settings"="Trigger Settings", "Handle In"=w18) -> ("error out"=w10:errorcluster, "Range"=w25:u16, "handle out"=w11:i16)  [unwired: 4 in]
  n76 = Obtain Queue(element data type=i16[][] [] ("buffer")) -> (queue out=w1:refnum<queue>, error out=w29:errorcluster)  [unwired: 4 in, 1 out]
  n77 = call "picoSetMem.vi"("error in (no error)"=w10, "Rapid Block Acquisition Settings"="Rapid Block Acquisition Settings", "Handle In"=w11) -> ("timebase"=w8:u32, "postTriggerSamples"=w7:u32, "Handle Out"=w6:i16, "nCaptures"=w9:u16)  [unwired: 4 in, 1 out]
  n78 = call "picoExtractSettings.vi"("Rapid Block Acquisition Settings"="Rapid Block Acquisition Settings") -> ("Down-Sample Mode"=w15:i32, "Down Sample Ratio"=w14:u32, "Numeric"=w13:i32)  [unwired: 8 in]
  n79 = while {
    tunnel: w6 -> [w200]
    tunnel: w7 -> [w199]
    tunnel: w8 -> [w198]
    tunnel: w9 -> [w204]
    tunnel: w13 -> [w196]
    tunnel: w14 -> [w195]
    tunnel: w15 -> [w194]
    tunnel: [w189] -> w28
    shift-right: [w186] -> _
    shift-left: w1 -> [w187]
    shift-right: [w184] -> w2
    shift-left: w29 -> [w183]
    stop <- w193 stop-if-true
    # "CRD Acquisition Loop (Producer)"
    n80 = call "picoRunBlock.vi"("error in (no error)"=w183, "timebase"=w198, "postTriggerSamples"=w199, "Handle In"=w200) -> ("error out"=w203:errorcluster, "handle"=w202:i16)  [unwired: 5 in, 1 out]
    n81 = call "picoReady.vi"("error in (no error)"=w203, "handle in"=w202) -> ("error out"=w201:errorcluster, "handle out"=w197:i16)  [unwired: 8 in]
    n82 = call "picoGetValues.vi"("Down-Sample Mode"=w194, "Down Sample Ratio"=w195, "nCaptures"=w204, "error in (no error)"=w201, "postTriggerSamples"=w196, "Handle In"=w197) -> ("error out"=w185:errorcluster, "buffer"=w188:i16[][], "handle"=w189:i16)  [unwired: 3 in]
    n83 = local read "Exit"() -> (w191:bool)
    n84 = Enqueue Element(queue=w187, element=w188, error in (no error)=w185) -> (queue out=w186:refnum<queue>, error out=w184:errorcluster)  [unwired: 1 in, 1 out]
    n85 = Unbundle By Name(w184) -> ("status"=w192:bool)
    n86 = Or(x=w192, y=w191) -> (x .or. y?=w193:bool)
    n87 = Wait (ms)(milliseconds to wait="crd delay") -> ()  [unwired: 1 out]
  }
  "error out" <- w2
  n88 = call <userlib>:"WaveIO_Stop.vi"("error in (no error)"=w68, "Handle"=w69) -> ("error out"=w70:errorcluster, "Handle Out"=w71:T9)
  n89 = Release Queue(queue=w83, error in (no error)=w84) -> (error out=w80:errorcluster)  [unwired: 1 in, 2 out]
  n90 = call <userlib>:"WaveIO_Stop.vi"("error in (no error)"=w66, "Handle"=w65) -> ("error out"=w64:errorcluster, "Handle Out"=w63:T9)
  n91 = Release Queue(queue=w55, error in (no error)=w54) -> (error out=w53:errorcluster)  [unwired: 1 in, 2 out]
  n92 = call <userlib>:"WaveIO_Close.vi"("error in (no error)"=w70, "Handle"=w71) -> ("error out"=w67:errorcluster)  [unwired: 1 out]
  n93 = call <userlib>:"WaveIO_Close.vi"("error in (no error)"=w64, "Handle"=w63) -> ("error out"=w52:errorcluster)  [unwired: 1 out]
  n94 = Divide(x=1.0, y=44100.0) -> (x/y=w44:dbl)
  n95 = Merge Errors(w67, w80, w52, w53) -> (w79:errorcluster)
  n96 = Obtain Queue(element data type=cluster{dbl, dbl, dbl} {0.0, 0.0, 0.0}) -> (queue out=w32:refnum<queue>, error out=w37:errorcluster)  [unwired: 4 in, 1 out]
  n97 = Obtain Queue(element data type=cluster{dbl, dbl, dbl} {0.0, 0.0, 0.0}) -> (queue out=w31:refnum<queue>, error out=w40:errorcluster)  [unwired: 4 in, 1 out]
  n98 = while "Message Processor" {
    shift-left: w93 -> [w219]
    shift-right: [w211] -> w89
    tunnel: w78 -> [w218]
    shift-left: "State Variables" -> [w224]
    shift-right: [w223] -> _
    tunnel: "320 Port" -> [w215]
    tunnel: "375 Port" -> [w214]
    tunnel: "445 Port" -> [w213]
    tunnel: "Teensy Port" -> [w212]
    shift-right: [w209] -> _
    shift-left: _ -> [w208]
    tunnel: w30 -> [w206]
    tunnel: "Chopper Port" -> [w205]
    stop <- w222 stop-if-true
    w216 = 100  # Timeout
    n99 = call "QMH Get Next Message from Queue.vi"("error in (no error)"=w219, "ms timeout (1)"=w216, "queue in"=w218) -> ("error out"=w220:errorcluster, "Next Parameter"=w207:string, "Next Message"=w217:string, "queue out"=w221:refnum<queue>, "Stop QMH"=w222:bool)  [unwired: 3 in]
    n100 = case shown="\"namefiles\"" w217 {
      selector: w217 -> [_ w253 _ _ _ _ _ _ _ _ _ _ _ _ _ _ _ _ _ _ _]
      tunnel: [w249 w254 w274 w284 w345 w368 w406 w435 w441 w447 w454 w461 w468 w488 w495 w519 w531 w548 w591 w597 w614] -> w223
      tunnel: w224 -> [w249 w254 w274 w284 w345 w368 w406 w435 w441 w447 w454 w461 w468 w488 w495 w519 w531 w548 w591 w597 w614]
      tunnel: w221 -> [_ _ _ w277 _ _ _ _ _ _ _ _ _ _ _ _ _ _ _ w595 w615]
      tunnel: w220 -> [w242 w250 w262 w283 w343 w363 w403 w437 w443 w445 w451 w458 w466 w489 w492 w517 w530 w549 w588 w596 w616]
      tunnel: [w241 w250 w258 w276 w342 w365 w404 w433 w439 w445 w452 w459 w462 w489 w491 w516 w530 w549 w589 w593 w602] -> w211
      tunnel: w215 -> [w239 _ w273 w275 _ _ w405 _ _ _ _ _ w465 _ _ _ _ _ _ _ w611]
      tunnel: w214 -> [w237 _ w271 w279 _ _ _ w434 _ _ w453 _ w464 _ _ _ _ _ _ _ w610]
      tunnel: w213 -> [w238 _ w270 w282 _ _ _ _ w440 _ _ w460 w463 _ _ _ _ _ _ _ w609]
      tunnel: w212 -> [_ _ w268 w278 w344 w366 _ _ _ _ _ _ _ _ w493 w518 _ _ _ _ w612]
      tunnel: w207 -> [_ _ _ _ w341 w361 _ _ _ _ w448 w455 _ _ _ w515 w529 _ _ _ _]
      tunnel: w206 -> [_ _ _ _ _ _ _ _ _ _ _ _ _ _ _ _ w528 _ _ _ _]
      tunnel: w205 -> [_ _ w263 _ _ _ w401 _ _ _ _ _ _ _ _ _ _ _ w590 _ w604]
      frame "", "Wait" {
        # "Update the front panel"
        # "Idle Case - this case is called after a Timeout on the Get Next Message from Queue VI, if no new messages are present on the queue. This case can be used for housekeeping tasks such as updating the UI."
        n101 = Get Date/Time String(want seconds? (F)=TRUE) -> (date string=w248:string, time string=w247:string)  [unwired: 2 in]
        n102 = call-poly "laserDiagnose.vi"("320 Port"=w239, "375 Port in"=w237, "445 Port 3"=w238, "error in (no error)"=w242) -> ("Powers"=→"Laser Powers":T10, "Currents"=→"Laser Currents":T11, "Temperatures"=→"Laser Temperatures":T2, "Overtemp"=→"Overtemp":bool, "error out"=w241:errorcluster)  [unwired: 7 in]
        n103 = Concatenate Strings(w248, " " ("string"), w247) -> (→"Status":string)
      }
      frame Default {
        # "Call this case if a message is received that is not handled \nby any other case. Typically this is a programming error\nas a result of a typo or unhandled message/missing message handler."
        n104 = Format Into String(format string="DevError: Missing message handler for '%s\" message." ("message"), w253) -> (resulting string=w251:string)  [unwired: 2 in, 1 out]
        n105 = One Button Dialog(message=w251) -> ()  [unwired: 1 in, 1 out]
      }
      frame "Initialize" {
        w255 = u16 1 items=["stop", "start", "ask"] ("start/stop")
        w264 = u32 115200 ("baud rate (9600)")
        # "Initialize the state variables and user interface\nInitialize serial connections"
        n106 = call-poly "VISA Configure Serial Port"("VISA resource name"=w263, "baud rate (9600)"=w264, "error in (no error)"=w262) -> ("VISA resource name out"=w261:refnum<visa-resource-name>, "error out"=w260:errorcluster)  [unwired: 11 in]
        n107 = call-poly "VISA Configure Serial Port"("VISA resource name"=w273, "baud rate (9600)"=u32 19200, "error in (no error)"=w260) -> ("error out"=w272:errorcluster)  [unwired: 11 in, 1 out]
        n108 = call-poly "VISA Configure Serial Port"("VISA resource name"=w271, "baud rate (9600)"=w264, "error in (no error)"=w272) -> ("error out"=w269:errorcluster)  [unwired: 11 in, 1 out]
        n109 = call-poly "VISA Configure Serial Port"("VISA resource name"=w270, "baud rate (9600)"=w264, "error in (no error)"=w269) -> ("error out"=w267:errorcluster)  [unwired: 11 in, 1 out]
        n110 = call-poly "VISA Configure Serial Port"("VISA resource name"=w268, "error in (no error)"=w267) -> ("VISA resource name out"=w266:refnum<visa-resource-name>, "error out"=w265:errorcluster)  [unwired: 12 in]
        n111 = property class="Instr" props=["Baud"](reference=w266, error in=w265) -> (error out=w259:errorcluster)  [unwired: 2 out]
        n112 = call "chopperStartStop.vi"("error in (no error)"=w259, "start/stop"=w255, "VISA Refnum in"=w261) -> ("error out"=w258:errorcluster, "Chopper On?"=w256:bool)  [unwired: 6 in, 1 out]
        n113 = local write "Chopper On"(w256) -> ()
      }
      frame "sweep" {
        # "Perform a frequency sweep and calculate the resonance frequency"
        n114 = stacked-sequence {
          seq-local: [_ w301 _ _] -> [_ _ w329 _]
          tunnel: w283 -> [w290 w295 _ _]
          tunnel: "Data End Frequency (Hz)" -> [_ w298 w323 _]
          tunnel: "Data Start Frequency (Hz)" -> [_ w297 w322 _]
          tunnel: w282 -> [_ _ _ _]
          tunnel: w279 -> [w291 _ _ w336]
          tunnel: w278 -> [w285 w296 _ _]
          tunnel: w277 -> [_ _ _ w339]
          tunnel: [w288 _ _ _] -> w276
          tunnel: w275 -> [_ _ _ _]
          frame #0 {
            w287 = u16 0 items=["blue", "green", "red"] ("laser")
            # "Turn UV lasers off for scan."
            n115 = call "laserOnOff.vi"("error in (no error)"=w290, "Emission (F = OFF)"=FALSE, "VISA Refnum in"=w291) -> ("error out"=w289:errorcluster)  [unwired: 6 in, 2 out]
            n116 = Wait (ms)(milliseconds to wait=u32 5000) -> ()  [unwired: 1 out]
            n117 = local write "Status"("Conducting Frequency Sweep" ("Status")) -> ()
            n118 = call "freqSet.vi"("error in (no error)"=w289, "laser"=w287, "Freq, Hz (1370)"=1500, "Teensy Port"=w285) -> ("error out"=w288:errorcluster)  [unwired: 6 in, 1 out]
          }
          frame #1 {
            n119 = Subtract(x=w298, y=w297) -> (x-y=w299:i32)
            n120 = for {
              N: w299 -> [w305]
              tunnel: [w310] -> w301 mode=indexing
              tunnel: w297 -> [w309]
              tunnel: w298 -> [w308]
              tunnel: w295 -> [_]
              i -> [w302]
              # "Get microphone data."
              # "Listen for N*2000\n seconds"
              n121 = Increment(x=w302) -> (x+1=w303:i32)
              n122 = Divide(x=w303, y=w305) -> (x/y=→"sweep progress":dbl)
              n123 = local read "micfft"() -> (w307:cluster{"f0":dbl, "df":dbl, "magnitude":dbl[]})
              n124 = Unbundle By Name(w307) -> ("magnitude"=w306:dbl[])
              n125 = Wait (ms)(milliseconds to wait=u32 2000) -> ()  [unwired: 1 out]
              n126 = call "fftGetMax.vi"("End Frequency (Hz)"=w308, "Start Frequency (Hz)"=w309, "Magnitudes"=w306) -> ("max value"=w310:dbl)  [unwired: 8 in]
            }
            n127 = case shown="True" TRUE ("sweep?") {
              tunnel: w297 -> [_ w317]
              tunnel: w298 -> [_ w316]
              tunnel: w296 -> [_ w315]
              tunnel: [w312 w314] -> _
              tunnel: w295 -> [w312 w313]
              frame False {
              }
              frame True {
                # "Scan laser freq.\nwith Teensy"
                n128 = call "teensySweepFreq.vi"("error in (no error)"=w313, "end f, Hz (1385)"=w316, "start f, Hz (1355)"=w317, "VISA Refnum in"=w315) -> ("error out"=w314:errorcluster)  [unwired: 7 in]
              }
            }
          }
          frame #2 {
            # "Calculate resonance frequency;\ndisplay and save scan."
            n129 = Wait (ms)(milliseconds to wait=u32 5000) -> ()  [unwired: 1 out]
            n130 = local read "PAS Save"() -> (w318:bool)
            n131 = To Double Precision Float(number=w323) -> (double precision float=w320:dbl)
            n132 = To Double Precision Float(number=w322) -> (double precision float=w321:dbl)
            n133 = call "resCalc.vi"("Frequency Sweep"=w329, "Start F, Hz (1355)"=w322) -> ("F-res, Hz"=w327:dbl, "Frequency Scan"=w319:cluster{i32[], "Best Gaussian Fit":dbl[]}[])  [unwired: 8 in]
            "freqscan" <- w319
            n134 = In Range and Coerce(upper limit=w320, x=w327, lower limit=w321) -> (In Range?=w326:bool)  [unwired: 1 out]
            n135 = case shown="True" w318 {
              tunnel: w319 -> [_ w333]
              tunnel: w327 -> [_ w332]
              frame False {
              }
              frame True {
                n136 = local read "sweeps"() -> (w331:path)
                n137 = call "saveFreqSweep.vi"("f-res, Hz"=w332, "Frequency Scan"=w333, "file path (dialog if empty)"=w331) -> ()  [unwired: 9 in]
              }
            }
            n138 = And(x=w326, y=TRUE ("check freqs?")) -> (x .and. y?=w324:bool)
            n139 = case shown="True" w324 {
              tunnel: w327 -> [_ w330]
              frame False {
              }
              frame True {
                n140 = property on="Calculated Resonance (Hz)" class="DigNum (strict)"("Val(Sgnl)"=w330) -> ()  [unwired: 2 in, 2 out]
                "Calculated Resonance (Hz)" <- w330
              }
            }
          }
          frame #3 {
            # "Turn UV lasers back on."
            n141 = local read "375 Power (mW)"() -> (w335:dbl)
            n142 = call "laserOnOff.vi"("Emission (F = OFF)"=TRUE, "Power, mW (100)"=w335, "VISA Refnum in"=w336) -> ("error out"=w334:errorcluster)  [unwired: 6 in, 2 out]
            n143 = call-poly "QMH Add Message to Queue.vi"("error in (no error)"=w334, "Parameter"="532 F (Hz)", "Message"="freqset", "queue in"=w339) -> ()  [unwired: 6 in, 2 out]
          }
        }
      }
      frame "freqset" {
        # "Set the frequency of the Teensy's modulation\nsignal for single laser (if single frequency is changed)."
        # "Set the laser frequency.  Case for \"red\", \"blue\", or \"green\"."
        n144 = case shown="\"320 F (Hz) \", Default" w341 {
          tunnel: w343 -> [w350 w355 w360]
          tunnel: [w349 w354 w359] -> w342
          tunnel: w344 -> [w346 w351 w357]
          frame "320 F (Hz) ", Default {
            w348 = u16 0 items=["blue", "green", "red"] ("laser")
            n145 = call "freqSet.vi"("error in (no error)"=w350, "laser"=w348, "Freq, Hz (1370)"="320 F (Hz)", "Teensy Port"=w346) -> ("error out"=w349:errorcluster)  [unwired: 6 in, 1 out]
          }
          frame "375 F (Hz)" {
            w353 = u16 1 items=["blue", "green", "red"] ("laser")
            n146 = call "freqSet.vi"("error in (no error)"=w355, "laser"=w353, "Freq, Hz (1370)"="375 F (Hz)", "Teensy Port"=w351) -> ("error out"=w354:errorcluster)  [unwired: 6 in, 1 out]
          }
          frame "445 F (Hz)" {
            w356 = u16 2 items=["blue", "green", "red", "ir"] ("laser")
            n147 = call "freqSet.vi"("error in (no error)"=w360, "laser"=w356, "Freq, Hz (1370)"="445 F (Hz)", "Teensy Port"=w357) -> ("error out"=w359:errorcluster)  [unwired: 6 in, 1 out]
          }
        }
      }
      frame "setfreqs" {
        # "Set the frequency of the Teensy's modulation\nsignal for all lasers at once."
        # "Set laser frequencies to resonance frequency calculated in sweep."
        n148 = Scan From String(input string=w361, error in=w363) -> (error out=w362:errorcluster, output 1=w364:dbl)  [unwired: 3 in, 2 out]
        n149 = for {
          N: 3 -> [_]
          tunnel: [w374] -> w365
          tunnel: w362 -> [w373]
          tunnel: w366 -> [w370]
          tunnel: w364 -> [w372]
          i -> [w371]
          n150 = flat-sequence {
            tunnel: w370 -> [w375]
            tunnel: [w375] -> w369
            frame #0 {
              n151 = Wait (ms)(milliseconds to wait=u32 1000) -> ()  [unwired: 1 out]
            }
          }
          n152 = case shown="0" w371 {
            tunnel: [w382 w390 w398] -> w374
            tunnel: w373 -> [w380 w387 w395]
            tunnel: w369 -> [w379 w386 w394]
            tunnel: w372 -> [w377 w383 w391]
            frame 0 {
              w381 = u16 2 items=["blue", "green", "red"] ("laser")
              n153 = To Long Integer(number=w377) -> (32bit integer=w378:i32)
              n154 = local write "445 F (Hz)"(w378) -> ()
              n155 = call "freqSet.vi"("error in (no error)"=w380, "laser"=w381, "Freq, Hz (1370)"=w378, "Teensy Port"=w379) -> ("error out"=w382:errorcluster)  [unwired: 6 in, 1 out]
            }
            frame 1, Default {
              w389 = u16 1 items=["blue", "green", "red"] ("laser")
              n156 = Add(x=w383, y=2.0) -> (x+y=w385:dbl)
              n157 = To Long Integer(number=w385) -> (32bit integer=w384:i32)
              n158 = call "freqSet.vi"("error in (no error)"=w387, "laser"=w389, "Freq, Hz (1370)"=w384, "Teensy Port"=w386) -> ("error out"=w390:errorcluster)  [unwired: 6 in, 1 out]
              n159 = local write "375 F (Hz)"(w384) -> ()
            }
            frame 2 {
              w397 = u16 0 items=["blue", "green", "red"] ("laser")
              n160 = Subtract(x=w391, y=2.0) -> (x-y=w393:dbl)
              n161 = To Long Integer(number=w393) -> (32bit integer=w392:i32)
              n162 = call "freqSet.vi"("error in (no error)"=w395, "laser"=w397, "Freq, Hz (1370)"=w392, "Teensy Port"=w394) -> ("error out"=w398:errorcluster)  [unwired: 6 in, 1 out]
              n163 = local write "320 F (Hz)"(w392) -> ()
            }
          }
        }
      }
      frame "320 emit" {
        w402 = u16 2 items=["stop", "start", "ask"] ("start/stop")
        n164 = call "chopperStartStop.vi"("error in (no error)"=w403, "start/stop"=w402, "VISA Refnum in"=w401) -> ("error out"=w399:errorcluster, "Chopper On?"=w400:bool)  [unwired: 6 in, 1 out]
        n165 = case shown="False" w400 {
          tunnel: w405 -> [_ w412]
          tunnel: [w408 w411] -> w404
          tunnel: w399 -> [w408 w409]
          frame False {
            n166 = One Button Dialog(message="Turn on chopper first!") -> ()  [unwired: 1 in, 1 out]
          }
          frame True {
            # "Turn laser on or off"
            n167 = case shown="False" "320 Emission" {
              tunnel: [w417 w425] -> w411
              tunnel: [w418 w426] -> _
              tunnel: w412 -> [w414 w423]
              tunnel: w409 -> [w413 w424]
              frame False {
                n168 = VISA Write(VISA resource name=w414, write buffer="45181\t3\t1030\r", error in (no error)=w413) -> (VISA resource name out=w415:refnum<visa-resource-name>, error out=w416:errorcluster)  [unwired: 1 out]
                n169 = property class="Instr"(reference=w415, error in=w416) -> (reference out=w419:refnum<visa-resource-name>, error out=w420:errorcluster, "Bytes at Port"=w421:u32)
                n170 = VISA Read(VISA resource name=w419, byte count=w421, error in (no error)=w420) -> (VISA resource name out=w418:refnum<visa-resource-name>, error out=w417:errorcluster)  [unwired: 2 out]
              }
              frame True {
                n171 = VISA Write(VISA resource name=w423, write buffer="33612\t3\t1020\r", error in (no error)=w424) -> (VISA resource name out=w428:refnum<visa-resource-name>, error out=w427:errorcluster)  [unwired: 1 out]
                n172 = property class="Instr"(reference=w428, error in=w427) -> (reference out=w431:refnum<visa-resource-name>, error out=w430:errorcluster, "Bytes at Port"=w429:u32)
                n173 = VISA Read(VISA resource name=w431, byte count=w429, error in (no error)=w430) -> (VISA resource name out=w426:refnum<visa-resource-name>, error out=w425:errorcluster)  [unwired: 2 out]
              }
            }
          }
        }
      }
      frame "375 emit" {
        # "Turn laser on or off"
        n174 = call "laserOnOff.vi"("error in (no error)"=w437, "Emission (F = OFF)"="375 Emission", "Power, mW (100)"="375 Power (mW)", "VISA Refnum in"=w434) -> ("error out"=w433:errorcluster)  [unwired: 5 in, 2 out]
      }
      frame "445 emit" {
        # "Turn laser on or off"
        n175 = call "laserOnOff.vi"("error in (no error)"=w443, "Emission (F = OFF)"="445 Emission", "Power, mW (100)"="445 Power (mW)", "VISA Refnum in"=w440) -> ("error out"=w439:errorcluster)  [unwired: 5 in, 2 out]
      }
      frame "emit" {
        # "Turn on all lasers."
        n176 = local write "320 Emission"("All Emit") -> ()
        n177 = local write "375 Emission"("All Emit") -> ()
        n178 = local write "445 Emission"("All Emit") -> ()
      }
      frame "532 Power" {
        n179 = Scan From String(input string=w448, error in=w451) -> (error out=w450:errorcluster, output 1=w449:dbl)  [unwired: 3 in, 2 out]
        n180 = call "laserSetPower.vi"("error in (no error)"=w450, "Laser Power (mW)"=w449, "VISA Refnum in"=w453) -> ("error out"=w452:errorcluster)  [unwired: 7 in, 1 out]
      }
      frame "782 Power" {
        n181 = Scan From String(input string=w455, error in=w458) -> (error out=w457:errorcluster, output 1=w456:dbl)  [unwired: 3 in, 2 out]
        n182 = call "laserSetPower.vi"("error in (no error)"=w457, "Laser Power (mW)"=w456, "VISA Refnum in"=w460) -> ("error out"=w459:errorcluster)  [unwired: 7 in, 1 out]
      }
      frame "align" {
        # "Set power of all lasers to 5 mW for alignment"
        n183 = case shown="False" "Alignment Mode" {
          tunnel: w466 -> [w476 w485]
          tunnel: w465 -> [w475 w484]
          tunnel: w464 -> [w474 w483]
          tunnel: w463 -> [w473 w482]
          tunnel: [w470 w479] -> w462
          frame True {
            w469 = 5.0 ("Laser Power (mW)")
            n184 = call "laserSetPower.vi"("error in (no error)"=w476, "Laser Power (mW)"=w469, "VISA Refnum in"=w475) -> ("error out"=w472:errorcluster)  [unwired: 7 in, 1 out]
            n185 = call "laserSetPower.vi"("error in (no error)"=w472, "Laser Power (mW)"=w469, "VISA Refnum in"=w474) -> ("error out"=w471:errorcluster)  [unwired: 7 in, 1 out]
            n186 = call "laserSetPower.vi"("error in (no error)"=w471, "Laser Power (mW)"=w469, "VISA Refnum in"=w473) -> ("error out"=w470:errorcluster)  [unwired: 7 in, 1 out]
          }
          frame False, Default {
            n187 = local read "375 Power (mW)"() -> (w478:dbl)
            n188 = local read "445 Power (mW)"() -> (w477:dbl)
            n189 = call "laserSetPower.vi"("error in (no error)"=w485, "VISA Refnum in"=w484) -> ("error out"=w481:errorcluster)  [unwired: 8 in, 1 out]
            n190 = call "laserSetPower.vi"("error in (no error)"=w481, "Laser Power (mW)"=w478, "VISA Refnum in"=w483) -> ("error out"=w480:errorcluster)  [unwired: 7 in, 1 out]
            n191 = call "laserSetPower.vi"("error in (no error)"=w480, "Laser Power (mW)"=w477, "VISA Refnum in"=w482) -> ("error out"=w479:errorcluster)  [unwired: 7 in, 1 out]
          }
        }
      }
      frame "background" {
        n192 = local read "mic ts"() -> (w487:T7)
        n193 = local read "tau"() -> (w486:dbl)
        n194 = local write "Bkg Values (mV)"(w487) -> ()
        n195 = local write "tau0"(w486) -> ()
      }
      frame "filter" {
        n196 = local read "Filtering"() -> (w494:bool)
        n197 = case shown="True" w494 {
          tunnel: w493 -> [w498 w507]
          tunnel: w492 -> [w497 w505]
          tunnel: [w496 w506] -> w491
          frame False {
            n198 = Multiply(x="Filter Length (min)", y=60.0) -> (x*y=w501:dbl)
            n199 = local write "Time Target (s)"(w501) -> ()
            n200 = VISA Write(VISA resource name=w498, write buffer="v.1", error in (no error)=w497) -> (error out=w496:errorcluster)  [unwired: 2 out]
            "Filtering" <- TRUE
          }
          frame True {
            n201 = flat-sequence {
              tunnel: w505 -> [w513]
              tunnel: [w513] -> w504
              frame #0 {
                n202 = local read "mic ts"() -> (w514:T7)
                n203 = local write "Bkg Values (mV)"(w514) -> ()
              }
            }
            n204 = local write "Filtering"(FALSE) -> ()
            n205 = VISA Write(VISA resource name=w507, write buffer="v.0", error in (no error)=w504) -> (error out=w506:errorcluster)  [unwired: 2 out]
            n206 = Multiply(x="Sample Length (min)", y=60.0) -> (x*y=w509:dbl)
            n207 = local write "Time Target (s)"(w509) -> ()
          }
        }
        n208 = Wait (ms)(milliseconds to wait=u32 500) -> ()  [unwired: 1 out]
      }
      frame "filterswitch" {
        n209 = case shown="\"TRUE\"" w515 {
          tunnel: w518 -> [w522 w527]
          tunnel: w517 -> [w521 w526]
          tunnel: [w520 w525] -> w516
          frame "FALSE", Default {
            n210 = VISA Write(VISA resource name=w522, write buffer="v.0", error in (no error)=w521) -> (error out=w520:errorcluster)  [unwired: 2 out]
          }
          frame "TRUE" {
            n211 = VISA Write(VISA resource name=w527, write buffer="v.1", error in (no error)=w526) -> (error out=w525:errorcluster)  [unwired: 2 out]
          }
        }
      }
      frame "namefiles" {
        n212 = case shown="\"TRUE\"" w529 {
          tunnel: w528 -> [_ w533]
          frame "FALSE", Default {
            n213 = local write "PAS Save"(FALSE ("PAS Save")) -> ()
          }
          frame "TRUE" {
            n214 = flat-sequence {
              tunnel: [w539] -> w536
              tunnel: [w541] -> w535
              tunnel: w536 -> [w541]
              tunnel: w535 -> [w543]
              tunnel: w534 -> [w542]
              frame #0 {
                n215 = call "saveSetDirectory.vi"() -> ("working directory"=→"working directory":path, "pas"=w539:path, "sweeps"=→"sweeps":path)  [unwired: 10 in, 3 out]
                "pas" <- w539
              }
              frame #1 {
                "PAS Save" <- TRUE ("PAS Save")
              }
              frame #2 {
                n216 = call-poly <vilib>:"Write To Spreadsheet File.vi"("append to file? (new file:F)"=TRUE, "2D data"=w542, "file path (dialog if empty)"=w543) -> ()  [unwired: 5 in, 1 out]
              }
            }
            n217 = Build Array(w533) -> (w534:string[][])
          }
        }
      }
      frame "savespec" {
        w545 = -1
        w581 = TRUE ("append to file? (new file:F)")
        n218 = local read "Filtering"() -> (w552:bool)
        n219 = local read "mic ts"() -> (w554:T7)
        n220 = local read "pd ts"() -> (w551:cluster{dbl, dbl, dbl})
        n221 = local read "tau"() -> (w546:dbl)
        n222 = Boolean To (0,1)(Boolean=w552) -> (0, 1=w560:i16)
        n223 = Unbundle(w554) -> ("422 Mean"=w567:dbl, "532 Mean"=w555:dbl, "785 Mean"=w556:dbl)
        n224 = Unbundle(w551) -> (w557:dbl, w558:dbl, w547:dbl)
        n225 = Format Date/Time String(time format string (%c)="%Y-%m-%d %H:%M:%S\t") -> (date/time string=w559:string)  [unwired: 2 in]
        n226 = Format Into String(w560) -> (resulting string=w561:string)  [unwired: 3 in, 1 out]
        n227 = Build Array(320, 375, 445) -> (w571:i32[])
        n228 = Build Array(w567, w555, w556) -> (w562:dbl[])
        n229 = Build Array(w557, w558, w547) -> (w550:dbl[])
        n230 = Build Array(w545, w545, w546) -> ()  [unwired: 1 out]
        n231 = Build Array(w559, w561) -> (w576:string[])
        n232 = Build Array(string[] ["wavelength_nm", "mic_mV", "PD_mW", ""]) -> (w580:string[][])
        n233 = Build Array(w571, w562, w550) -> (w565:dbl[][])
        n234 = Build Array(w576) -> (w577:string[][])
        n235 = Transpose 2D Array(2D array=w565) -> (transposed array=w566:dbl[][])
        n236 = Array To Spreadsheet String(array=w566, 3:"%.4e") -> (spreadsheet string=w572:string)  [unwired: 1 in]
        n237 = call-poly <vilib>:"Write To Spreadsheet File.vi"("transpose? (no:F)"=TRUE, "append to file? (new file:F)"=w581, "2D data"=w577) -> ("new file path (Not A Path if cancelled)"=w579:path)  [unwired: 5 in]
        n238 = Build Array(w572) -> (w583:string[])
        n239 = call-poly <vilib>:"Write To Spreadsheet File.vi"("transpose? (no:F)"=FALSE, "append to file? (new file:F)"=w581, "2D data"=w580, "file path (dialog if empty)"=w579) -> ("new file path (Not A Path if cancelled)"=w582:path)  [unwired: 4 in]
        n240 = call-poly <vilib>:"Write To Spreadsheet File.vi"("delimiter (\\t)"="" ("delimiter (\\t)"), "transpose? (no:F)"=FALSE, "append to file? (new file:F)"=TRUE, "1D data"=w583, "file path (dialog if empty)"=w582) -> ()  [unwired: 3 in, 1 out]
      }
      frame "chopper enable" {
        n241 = Boolean To (0,1)(Boolean="Chopper") -> (0, 1=w586:i16)
        n242 = call "chopperStartStop.vi"("error in (no error)"=w588, "start/stop"=w586, "VISA Refnum in"=w590) -> ("error out"=w589:errorcluster, "Chopper On?"=→"Chopper On":bool)  [unwired: 6 in, 1 out]
      }
      frame "Error" {
        (unwired) errorcluster {"status"=FALSE, "code"=0, "source"=""} ("error out")
        # "Proceed to Exit - remove if this is\nnot appropriate for the General Error case"
        # "General Error Case - this case is called if an error is passed using the error cluster below. Typically most new errors should be handed in each individual case and not passed in the rror cluster. If necessary a custom error handler case should be added and called from other cases."
        n243 = call <vilib>:"Simple Error Handler.vi"("error in (no error)"=w596) -> ("error out"=w592:errorcluster)  [unwired: 4 in, 4 out]
        n244 = call-poly "QMH Add Message to Queue.vi"("error in (no error)"=w592, "Message"="Exit", "queue in"=w595) -> ("error out"=w593:errorcluster)  [unwired: 7 in, 1 out]
      }
      frame "Exit" {
        w601 = u16 0 items=["stop", "start", "ask"] ("start/stop")
        # "Perform cleanup tasks: Close serial connections and clear front panel."
        n245 = call "QMH Destroy Queue.vi"("error in (no error)"=w616, "queue in"=w615) -> ("error out"=w608:errorcluster)  [unwired: 7 in, 2 out]
        n246 = for {
          N: 3 -> [_]
          tunnel: w611 -> [w623]
          tunnel: w610 -> [w621]
          tunnel: w609 -> [w620]
          tunnel: w608 -> [w619]
          tunnel: FALSE -> [w618]
          tunnel: [w617] -> w605
          i -> [w622]
          # "Close laser serial connections."
          n247 = case shown="0, Default" w622 {
            tunnel: [w630 w635 w640] -> w625
            tunnel: [w629 w634 w639] -> w624
            tunnel: w623 -> [w628 _ _]
            tunnel: w621 -> [_ w633 _]
            tunnel: w620 -> [_ _ w637]
            tunnel: w619 -> [w627 w632 w638]
            tunnel: w618 -> [w626 w631 w636]
            frame 0, Default {
              n248 = call "laserOnOff.vi"("error in (no error)"=w627, "Emission (F = OFF)"=w626, "VISA Refnum in"=w628) -> ("error out"=w630:errorcluster, "VISA Refnum out"=w629:refnum<visa-resource-name>)  [unwired: 6 in, 1 out]
              n249 = local write "320 Emission"(w626) -> ()
            }
            frame 1 {
              n250 = call "laserOnOff.vi"("error in (no error)"=w632, "Emission (F = OFF)"=w631, "VISA Refnum in"=w633) -> ("error out"=w635:errorcluster, "VISA Refnum out"=w634:refnum<visa-resource-name>)  [unwired: 6 in, 1 out]
              n251 = local write "375 Emission"(w631) -> ()
            }
            frame 2 {
              n252 = call "laserOnOff.vi"("error in (no error)"=w638, "Emission (F = OFF)"=w636, "VISA Refnum in"=w637) -> ("error out"=w640:errorcluster, "VISA Refnum out"=w639:refnum<visa-resource-name>)  [unwired: 6 in, 1 out]
              n253 = local write "445 Emission"(w636) -> ()
              n254 = local write "All Emit"(w636) -> ()
            }
          }
          n255 = VISA Close(VISA resource name=w624, error in (no error)=w625) -> (error out=w617:errorcluster)
        }
        n256 = local write "Status"("" ("Status")) -> ()
        n257 = VISA Close(VISA resource name=w612, error in (no error)=w605) -> (error out=w603:errorcluster)
        n258 = call "chopperStartStop.vi"("error in (no error)"=w603, "start/stop"=w601, "VISA Refnum in"=w604) -> ("error out"=w600:errorcluster, "Chopper On?"=w598:bool, "VISA Refnum out"=w599:refnum<visa-resource-name>)  [unwired: 6 in]
        n259 = local write "Chopper On"(w598) -> ()
        n260 = VISA Close(VISA resource name=w599, error in (no error)=w600) -> (error out=w602:errorcluster)
      }
    }
    n261 = case shown="True" "Auto Filter" {
      tunnel: [w225 w227] -> w209
      tunnel: w208 -> [w225 w226]
      frame False {
      }
      frame True {
        # "This is the timer for the filtering routine."
        n262 = call "Elapsed Time"("Time Target (s)"="Time Target (s)", "Auto Reset"=TRUE, "error in (no error)"=w226) -> ("Elapsed Time (s)"=w230:dbl, "Time has Elapsed"=w232:bool, "error out"=w231:errorcluster)  [unwired: 9 in, 5 out]
        "Time has Elapsed" <- w232
        n263 = Divide(x=w230, y=60.0) -> (x/y=→"Elapsed Time (min)":dbl)
        n264 = property on="Time has Elapsed" class="Bool (strict)"(error in=w231, "Val(Sgnl)"=w232) -> (error out=w227:errorcluster)  [unwired: 1 in, 1 out]
      }
    }
  }
  n265 = while {
    tunnel: w43 -> [w657]
    shift-right: [w654] -> _
    shift-left: w81 -> [w651]
    shift-right: [w653] -> _
    shift-left: w81 -> [w650]
    shift-right: [w652] -> _
    shift-left: w81 -> [w649]
    tunnel: w44 -> [w647]
    tunnel: "mic cal, scu" -> [w646]
    shift-right: [w644] -> w39
    shift-left: w31 -> [w643]
    shift-right: [w641] -> w38
    shift-left: w40 -> [w645]
    stop <- w648 stop-if-true
    # "Microphone Processing Loop (Consumer)"
    n266 = Dequeue Element(queue=w657) -> (element=w655:i32[][], error out=w656:errorcluster)  [unwired: 2 in, 2 out]
    n267 = case shown="No Error" w656 {
      selector: w656 -> [_ w688]
      tunnel: w655 -> [w681 _]
      tunnel: w651 -> [w685 w691]
      tunnel: w650 -> [w684 w689]
      tunnel: w649 -> [w683 w690]
      tunnel: [w661 w691] -> w654
      tunnel: [w660 w689] -> w653
      tunnel: [w659 w690] -> w652
      tunnel: [w658 w688] -> w648
      tunnel: w647 -> [w679 _]
      tunnel: w646 -> [w673 _]
      tunnel: [w662 T12 {"405 Mean"=0.0, "532 Mean"=0.0, "660 Mean"=0.0}] -> w642
      frame No Error {
        w686 = T13 0 items=["Rectangle"=0, "Hanning"=1, "Hamming"=2, "Blackman-Harris"=3, "Exact Blackman"=4, "Blackman"=5, "Flat Top"=6, "4 Term B-Harris "=7, "7 Term B-Harris"=8, "Low Sidelobe"=9, "Blackman Nuttall"=11, "Triangle"=30, "Bartlett-Hanning"=31, "Bohman"=32, "Parzen"=33, "Welch"=34, "Kaiser"=60, "Dolph-Chebyshev"=61, "Gaussian"=62] ("window")
        n268 = Index Array(array=w681, index (row)=0) -> (element=w680:i32[])  [unwired: 1 in]
        n269 = Bundle By Name("Y"=w680, "dt"=w679) -> (w678:waveform(i32))  [unwired: 1 in]
        "micwave" <- w678
        n270 = local read "320 F (Hz)"() -> (w676:i32)
        n271 = local read "375 F (Hz)"() -> (w675:i32)
        n272 = local read "445 F (Hz)"() -> (w674:i32)
        n273 = call-poly <vilib>:"FFT Spectrum (Mag-Phase).vi"("window"=w686, "time signal"=w678) -> ("error out"=w658:errorcluster, "magnitude"=w677:cluster{"f0":dbl, "df":dbl, "magnitude":dbl[]})  [unwired: 5 in, 3 out]
        "micfft" <- w677
        n274 = call-poly "fftGetMagsPoly.vi"("input cluster"=w677, "422 F (Hz)"=w676, "532 F (Hz)"=w675, "785 F (Hz)"=w674, "unit cal, scu"=w673) -> ("mag422 (mV)"=w668:dbl, "mag532 (mV)"=w667:dbl, "mag785 (mV)"=w666:dbl)  [unwired: 8 in]
        n275 = Bundle("X"=w685, "mag422 (mV)"=w668) -> (w672:cluster{"X":dbl[], "mag422 (mV) ":dbl})  [unwired: 1 in]
        n276 = Bundle("X"=w684, "mag532 (mV)"=w667) -> (w671:cluster{"X":dbl[], "mag532 (mV)":dbl})  [unwired: 1 in]
        n277 = Bundle("X"=w683, "mag785 (mV)"=w666) -> (w670:cluster{"X":dbl[], "mag785 (mV)":dbl})  [unwired: 1 in]
        n278 = call-poly "rollingAverage_multi.vi"("Magnitude Averaging (no. Avgs.)"="rollavg", "785nm"=w670, "532nm"=w671, "422nm"=w672) -> ("785nm Data"=w663:T14, "532nm Data"=w664:T15, "422nm Data"=w665:T16)  [unwired: 5 in]
        n279 = call-poly "micUnbundle.vi"("422nm Data"=w665, "532nm Data"=w664, "785nm Data"=w663) -> ("Output Cluster"=w662:T7, "422 New Array"=w661:dbl[], "532 New Array"=w660:dbl[], "785 New Array"=w659:dbl[])  [unwired: 9 in]
        "mic ts" <- w662
      }
      frame Error {
      }
    }
    n280 = Enqueue Element(queue=w643, element=w642, error in (no error)=w645) -> (queue out=w644:refnum<queue>, error out=w641:errorcluster)  [unwired: 1 in, 1 out]
  }
  n281 = while {
    shift-right: [w709] -> _
    shift-left: w81 -> [w706]
    shift-right: [w708] -> _
    shift-left: w81 -> [w705]
    shift-right: [w707] -> _
    shift-left: w81 -> [w704]
    tunnel: w47 -> [w702]
    tunnel: w44 -> [w701]
    tunnel: "mic cal, scu" -> [w700]
    shift-right: [w697] -> w36
    shift-left: w32 -> [w698]
    shift-right: [w696] -> w35
    shift-left: w37 -> [w699]
    stop <- w703 stop-if-true
    # "Photodiode Processing Loop (Consumer)"
    n282 = Dequeue Element(queue=w702) -> (element=w710:i32[][], error out=w711:errorcluster)  [unwired: 2 in, 2 out]
    n283 = case shown="No Error" w711 {
      selector: w711 -> [_ w745]
      tunnel: w710 -> [w738 _]
      tunnel: w706 -> [w742 w748]
      tunnel: w705 -> [w741 w746]
      tunnel: w704 -> [w740 w747]
      tunnel: [w719 w748] -> w709
      tunnel: [w718 w746] -> w708
      tunnel: [w717 w747] -> w707
      tunnel: [w713 w745] -> w703
      tunnel: w701 -> [w736 _]
      tunnel: w700 -> [w730 _]
      tunnel: "660 PD Cal 3" -> [w714 _]
      tunnel: "532 PD Cal 3" -> [w715 _]
      tunnel: "405 PD Cal 3" -> [w716 _]
      tunnel: [w712 cluster{dbl, dbl, dbl} {0.0, 0.0, 0.0}] -> w695
      frame No Error {
        w743 = T13 0 items=["Rectangle"=0, "Hanning"=1, "Hamming"=2, "Blackman-Harris"=3, "Exact Blackman"=4, "Blackman"=5, "Flat Top"=6, "4 Term B-Harris "=7, "7 Term B-Harris"=8, "Low Sidelobe"=9, "Blackman Nuttall"=11, "Triangle"=30, "Bartlett-Hanning"=31, "Bohman"=32, "Parzen"=33, "Welch"=34, "Kaiser"=60, "Dolph-Chebyshev"=61, "Gaussian"=62] ("window")
        n284 = Index Array(array=w738, index (row)=0) -> (element=w737:i32[])  [unwired: 1 in]
        n285 = Bundle By Name("Y"=w737, "dt"=w736) -> (w735:waveform(i32))  [unwired: 1 in]
        "pdwave" <- w735
        n286 = local read "320 F (Hz)"() -> (w733:i32)
        n287 = local read "375 F (Hz)"() -> (w732:i32)
        n288 = local read "445 F (Hz)"() -> (w731:i32)
        n289 = call-poly <vilib>:"FFT Spectrum (Mag-Phase).vi"("window"=w743, "time signal"=w735) -> ("error out"=w713:errorcluster, "magnitude"=w734:cluster{"f0":dbl, "df":dbl, "magnitude":dbl[]})  [unwired: 5 in, 3 out]
        "pdfft" <- w734
        n290 = call-poly "fftGetMagsPoly.vi"("input cluster"=w734, "422 F (Hz)"=w733, "532 F (Hz)"=w732, "785 F (Hz)"=w731, "unit cal, scu"=w730) -> ("mag422 (mV)"=w725:dbl, "mag532 (mV)"=w724:dbl, "mag785 (mV)"=w723:dbl)  [unwired: 8 in]
        n291 = Bundle("X"=w742, "mag422 (mV)"=w725) -> (w729:cluster{"X":dbl[], "mag422 (mV) ":dbl})  [unwired: 1 in]
        n292 = Bundle("X"=w741, "mag532 (mV)"=w724) -> (w728:cluster{"X":dbl[], "mag532 (mV)":dbl})  [unwired: 1 in]
        n293 = Bundle("X"=w740, "mag785 (mV)"=w723) -> (w727:cluster{"X":dbl[], "mag785 (mV)":dbl})  [unwired: 1 in]
        n294 = call-poly "rollingAverage_multi.vi"("Magnitude Averaging (no. Avgs.)"="Chart Rolling Average", "785nm"=w727, "532nm"=w728, "422nm"=w729) -> ("785nm Data"=w720:T14, "532nm Data"=w721:T15, "422nm Data"=w722:T16)  [unwired: 5 in]
        n295 = call-poly "pdNormalize.vi"("422 Data"=w722, "532 Data"=w721, "785 Data"=w720, "422 PD Cal 3"=w716, "532 PD Cal 3"=w715, "785 PD Cal 3"=w714) -> ("pd ts"=w712:cluster{dbl, dbl, dbl}, "422 New Array"=w719:dbl[], "532 New Array"=w718:dbl[], "785 New Array"=w717:dbl[])  [unwired: 5 in, 1 out]
        "pd ts" <- w712
      }
      frame Error {
      }
    }
    n296 = Enqueue Element(queue=w698, element=w695, error in (no error)=w699) -> (queue out=w697:refnum<queue>, error out=w696:errorcluster)  [unwired: 1 in, 1 out]
  }
  n297 = while {
    tunnel: w32 -> [w750]
    tunnel: w31 -> [w749]
    stop <- w756 stop-if-true
    # "Absorption Data Loop (Consummer II)"
    n298 = Dequeue Element(queue=w749) -> (element=w757:cluster{dbl, dbl, dbl}, error out=w755:errorcluster)  [unwired: 2 in, 2 out]
    n299 = Dequeue Element(queue=w750) -> (element=w752:cluster{dbl, dbl, dbl}, error out=w754:errorcluster)  [unwired: 2 in, 2 out]
    n300 = Wait (ms)(milliseconds to wait="save interval (ms)") -> ()  [unwired: 1 out]
    n301 = Merge Errors(w755, w754) -> (w753:errorcluster)
    n302 = case shown="No Error" w753 {
      selector: w753 -> [w792 w797]
      tunnel: w757 -> [w769 _]
      tunnel: [w781 w797] -> w756
      tunnel: w752 -> [w766 _]
      frame No Error {
        w759 = 0.0
        n303 = local read "tau0"() -> (w762:dbl)
        n304 = local read "tau"() -> (w760:dbl)
        n305 = Bundle("tau"=w760, "tau0"=w762) -> (w761:cluster{"tau":dbl, "tau0":dbl})  [unwired: 1 in]
        n306 = call-poly "absCalcPlot.vi"("CRD t, t0"=w761, "Cell Calibration, mV/mW"="cellcal", "Error In"=w792, "PD Values"=w766, "bkg values"="Bkg Values (mV)", "Mic Values"=w769) -> ("Error Out"=w782:errorcluster, "aae"=→"AAE":dbl, "Time Series"=→"abs/ext":cluster{dbl, dbl, dbl, "b_ext (1/Mm)":dbl}, "Spectrum"=→"Absorption Spectrum":cluster{dbl[], "Best Power Fit":dbl[]}[])  [unwired: 2 in]
        n307 = local read "Elapsed Time (min)"() -> (w772:dbl)
        n308 = local read "Filtering"() -> (w775:bool)
        n309 = local read "abs/ext"() -> (w780:cluster{dbl, dbl, dbl, "b_ext (1/Mm)":dbl})
        n310 = local read "mic ts"() -> (w786:T7)
        n311 = local read "pd ts"() -> (w791:cluster{dbl, dbl, dbl})
        n312 = local read "Calculated Resonance (Hz)"() -> (w776:dbl)
        n313 = Boolean To (0,1)(Boolean=w775) -> (0, 1=w774:i16)
        n314 = Unbundle(w786) -> ("422 Mean"=w785:dbl, "532 Mean"=w784:dbl, "785 Mean"=w783:dbl)
        n315 = Unbundle(w791) -> (w787:dbl, w788:dbl, w789:dbl)
        n316 = Unbundle(w780) -> (w779:dbl, w778:dbl, w777:dbl, "b_ext (1/Mm)"=w763:dbl)
        n317 = To Double Precision Float(number=w774) -> (double precision float=w773:dbl)
        n318 = Format Into String(format string="%.4e\t%.4e\t%.4e\t%.4e\t%.4e\t%.4e\t%.4e\t%.4e\t%.4e\t%.4e\t%.4e\t%.4e\t%.4e\t%.4e\t%f\t%f\t%.1f", error in=w782, w785, w784, w783, w759, w787, w788, w789, w759, w760, w779, w778, w777, w759, w763, w776, w773, w772) -> (resulting string=w758:string, error out=w781:errorcluster)  [unwired: 1 in]
        "saveString" <- w758
        n319 = local read "PAS Save"() -> (w770:bool)
        n320 = case shown="True" w770 {
          tunnel: w758 -> [_ w794]
          frame False {
          }
          frame True {
            n321 = local read "pas"() -> (w793:path)
            n322 = Build Array(w794) -> (w796:string[])
            n323 = call-poly <vilib>:"Write To Spreadsheet File.vi"("append to file? (new file:F)"=TRUE, "1D data"=w796, "file path (dialog if empty)"=w793) -> ()  [unwired: 5 in, 1 out]
          }
        }
        n324 = local write "saveString"(w758) -> ()
      }
      frame Error {
      }
    }
  }
  n325 = call "PicoScope2000aClose.vi"("handle"=w28) -> ()  [unwired: 11 in]
  n326 = Release Queue(queue=w1, error in (no error)=w2) -> ()  [unwired: 1 in, 3 out]
  n327 = while {
    tunnel: w23 -> [w808]
    tunnel: w24 -> [w807]
    tunnel: w25 -> [w806]
    shift-right: [w805] -> _
    shift-left: _ -> [w804]
    tunnel: "factor" -> [w801]
    tunnel: w1 -> [w799]
    stop <- w802 stop-if-true
    # "CRD Processing Loop (Consumer)"
    n328 = Multiply(x=w808, y=w801) -> (x*y=w809:sgl)
    n329 = Dequeue Element(queue=w799, timeout in ms (-1)=1500) -> (element=w803:i16[][], error out=w800:errorcluster)  [unwired: 1 in, 2 out]
    n330 = case shown="No Error" w800 {
      selector: w800 -> [w821 w836]
      tunnel: w809 -> [w814 _]
      tunnel: w807 -> [w830 _]
      tunnel: w806 -> [w829 _]
      tunnel: [w828 w837] -> w805
      tunnel: w804 -> [w827 w837]
      tunnel: w803 -> [w826 _]
      tunnel: [w825 w836] -> w802
      frame No Error {
        w820 = 0
        n331 = call "picoCoAdd.vi"("error in (no error)"=w821, "Buffer In"=w826) -> ("error out"=w834:errorcluster, "Waveform Out"=w835:dbl[])  [unwired: 8 in]
        n332 = call "picoToVolts.vi"("error in (no error)"=w834, "Max_adc"=w830, "Range Index"=w829, "Data"=w835) -> ("error out"=w825:errorcluster, "Data (mV)"=w817:dbl[])  [unwired: 6 in]
        n333 = Array Subset(array=w817, index=0, length="N") -> (w816:dbl[])
        n334 = call "Get Tau.vi"("CalType"=analys_meth."DFT-5", "Dt"=w814, "X"=w816) -> ("B"=w822:dbl, "A"=w823:dbl, "tau"=w824:dbl)  [unwired: 5 in, 1 out]
        n335 = call "crdDisplayFit.vi"("dt"=w814, "N"="N", "B"=w822, "A"=w823, "tau"=w824) -> ("Fit Out"=w832:dbl[])  [unwired: 6 in]
        n336 = call "rollingAverage.vi"("No Avg"="tau Rolling Avg", "New Element"=w824, "Rolling Array"=w827) -> ("mean"=→"tau":dbl, "New Array"=w828:dbl[])  [unwired: 6 in, 1 out]
        n337 = Bundle(w820, w814, w816) -> (w813:cluster{i32, sgl, dbl[]})  [unwired: 1 in]
        n338 = Bundle(w820, w814, "Fit Out"=w832) -> (w812:cluster{i32, sgl, "Fit Out":dbl[]})  [unwired: 1 in]
        n339 = Subtract(x=w813, y=w812) -> (x-y=→"residual":cluster{i32, sgl, dbl[]})
        n340 = Build Array(w812, w813) -> (→"decay":cluster{i32, sgl, "Fit Out":dbl[]}[])
      }
      frame Error {
      }
    }
  }
  n341 = Release Queue(queue=w36, error in (no error)=w35) -> ()  [unwired: 1 in, 3 out]
  n342 = Release Queue(queue=w39, error in (no error)=w38) -> ()  [unwired: 1 in, 3 out]
  n343 = Merge Errors(w89, w79) -> (w88:errorcluster)
  n344 = while {
    stop <- w838 stop-if-true
    # "Spectrum Averaging & Saving Loop"
    n345 = case shown="True" "Save Average" {
      frame False {
      }
      frame True {
        w853 = TRUE ("transpose? (no:F)")
        n346 = local read "mic ts"() -> (w848:T7)
        n347 = local read "Filtering"() -> (w852:bool)
        n348 = local read "pd ts"() -> (w847:cluster{dbl, dbl, dbl})
        n349 = local read "tau"() -> (w846:dbl)
        n350 = call-poly "saveBuildHeader_poly.vi"("Filtering"=w852) -> ("wavelengths"=w850:string[], "header"=w851:string[])  [unwired: 9 in]
        n351 = for {
          N: "No. Averages" -> [_]
          tunnel: [w868] -> w845 mode=indexing
          tunnel: [w863] -> w844 mode=indexing
          tunnel: [w860] -> w843 mode=indexing
          tunnel: w848 -> [w859]
          tunnel: w847 -> [w858]
          tunnel: w846 -> [w857]
          w861 = 0.0 ("element")
          n352 = Unbundle(w859) -> ("422 Mean"=w869:dbl, "532 Mean"=w870:dbl, "785 Mean"=w866:dbl)
          n353 = Unbundle(w858) -> (w865:dbl, w864:dbl, w862:dbl)
          n354 = Build Array(w865, w864, w862) -> (w863:dbl[])
          n355 = Build Array(w861, w861, w857) -> (w860:dbl[])
          n356 = Build Array(w869, w870, w866) -> (w868:dbl[])
          n357 = Wait (ms)(milliseconds to wait=u32 1000) -> ()  [unwired: 1 out]
        }
        n358 = call "saveAvgSpectrum_III_BC.vi"("crd"=w843, "pd"=w844, "mic"=w845) -> ("CRD"=w841:string[], "PD"=w840:string[], "Mic"=w849:string[])  [unwired: 6 in]
        n359 = Build Array(w850, w849, w840, w841) -> (w855:string[][])
        n360 = call-poly <vilib>:"Write To Spreadsheet File.vi"("1D data"=w851) -> ("new file path (Not A Path if cancelled)"=w856:path)  [unwired: 7 in]
        n361 = call-poly <vilib>:"Write To Spreadsheet File.vi"("transpose? (no:F)"=w853, "append to file? (new file:F)"=w853, "2D data"=w855, "file path (dialog if empty)"=w856) -> ("new file path (Not A Path if cancelled)"=w854:path)  [unwired: 4 in]
        n362 = flat-sequence {
          tunnel: w854 -> [_]
          frame #0 {
            n363 = local write "Save Average"(FALSE ("append to file? (new file:F)")) -> ()
          }
        }
      }
    }
    n364 = local read "Exit"() -> (w838:bool)
  }
  n365 = call <vilib>:"Simple Error Handler.vi"("error in (no error)"=w88) -> ("error out"=w87:errorcluster)  [unwired: 4 in, 4 out]
  n366 = flat-sequence {
    tunnel: w87 -> [w872]
    tunnel: [w872] -> w86
    frame #0 {
      n367 = local write "Exit"(FALSE) -> ()
    }
  }
  "Error Console" <- w86
